vi "main 1.3.vi"() -> ()   [LabVIEW 2012]
uses:
  subvi/Newport ESP301/Newport ESP301.lvlib
  subvi/sp_manip.llb/sp_manip_lib.lvlib
  subvi/sp_manip.llb/tcp_gateway.lvlib
  subvi/PHOIBOS/DEFINITIONS/DEF_dev_type.ctl
  subvi/PHOIBOS/DEFINITIONS/DEF_dev_state.ctl
  <vilib>/Utility/file.llb/Write Delimited Spreadsheet (DBL).vi
  <vilib>/Analysis/NI_AALBase.lvlib
  <vilib>/Analysis/1siggen.llb/Ramp Pattern by Samples.vi
  <vilib>/Analysis/NI_AALPro.lvlib
  <vilib>/Analysis/_algsub.llb/Real Vector Norm.vi
  subvi/ZaberTSeries/ZaberTSeries.lvlib
  <vilib>/Utility/file.llb/Write Delimited Spreadsheet (string).vi
  <vilib>/Analysis/6fits.llb/Curve Fitting Criteria.ctl
  <vilib>/Instr/_visa.llb/VISA Configure Serial Port (Instr).vi
  <vilib>/DAQmx/create/channels.llb/DAQmx Create Channel (DI-Digital Input).vi
  <vilib>/Utility/file.llb/Read Delimited Spreadsheet (string).vi
panel:
  out "Pics L":i32=20
  out "Waveform Chart":dbl(graph)
  out "G2 X":cluster{dbl[], "Ramp Pattern":dbl[]}(graph)
  in  "reset every n pics":bool=TRUE
  in  "pics2avg":i32=50
  in  "abort acq.":bool
  out "G2 Y":cluster{dbl[], "Ramp Pattern":dbl[]}(graph)={[0.0, 0.0, 0.0, 0.0, 0.0, 0.0, 0.0, 0.0, 0.0, 0.0, 0.0, 0.0, 0.0, 0.0, 0.0, 0.0, 0.0, 0.0, 0.0, 0.0, 0.0, 0.0, 0.0, 0.0, 0.0, 0.0, 0.0, 0.0, 0.0, 0.0, 0.0, 0.0, 0.0, 0.0, 0.0, 0.0, 0.0, 0.0, 0.0, 0.0, 0.0, 0.0, 0.0, 0.0, 0.0, 0.0, 0.0, 0.0, 0.0, 0.0, 0.0, 0.0, 0.0, 0.0, 0.0, 0.0, 0.0, 0.0, 0.0, 0.0, 0.0, 0.0, 0.0, 0.0, 0.0, 0.0, 0.0, 0.0, 0.0, 0.0, 0.0, 0.0, 0.0, 0.0, 0.0, 0.0, 0.0, 0.0, 0.0, 0.0, 0.0, 0.0, 0.0, 0.0, 0.0, 0.0, 0.0, 0.0, 0.0, 0.0, 0.0, 0.0, 0.0, 0.0, 0.0, 0.0, 0.0, 0.0, 0.0, 0.0, 0.0, 0.0, 0.0, 0.0, 0.0, 0.0, 0.0, 0.0, 0.0, 0.0, 0.0, 0.0, 0.0, 0.0, 0.0, 0.0, 0.0, 0.0, 0.0, 0.0, 0.0, 0.0, 0.0, 0.0, 0.0, 0.0, 0.0, 0.0, 0.0, 0.0, 0.0, 0.0, 0.0, 0.0, 0.0, 0.0, 0.0, 0.0, 0.0, 0.0, 0.0, 0.0, 0.0, 0.0, 0.0, 0.0, 0.0, 0.0, 0.0, 0.0, 0.0, 0.0, 0.0, 0.0, 0.0, 0.0, 0.0, 0.0, 0.0, 0.0, 0.0, 0.0, 0.0, 0.0, 0.0, 0.0, 0.0, 0.0, 0.0, 0.0, 0.0, 0.0, 0.0, 0.0, 0.0, 0.0, 0.0, 0.0, 0.0, 0.0, 0.0, 0.0, 0.0, 0.0, 0.0, 0.0, 0.0, 0.0, 0.0, 0.0, 0.0, 0.0, 0.0, 0.0, 0.0, 0.0, 0.0, 0.0, 0.0, 0.0, 0.0, 0.0, 0.0, 0.0, 0.0, 0.0, 0.0, 0.0, 0.0, 0.0, 0.0, 0.0, 0.0, 0.0, 0.0, 0.0, 0.0, 0.0, 0.0, 0.0, 0.0, 0.0, 0.0, 0.0, 0.0, 0.0, 0.0, 0.0, 0.0, 0.0, 0.0, 0.0, 0.0, 0.0, 0.0, 0.0, 0.0, 0.0, 0.0, 0.0, 0.0, 0.0, 0.0, 0.0, 0.0, 0.0, 0.0, 0.0, 0.0, 0.0, 0.0, 0.0, 0.0, 0.0, 0.0, 0.0], "Ramp Pattern"=[0.0, 1.003921568627451, 2.007843137254902, 3.011764705882353, 4.015686274509804, 5.019607843137255, 6.023529411764706, 7.027450980392157, 8.031372549019608, 9.035294117647059, 10.03921568627451, 11.04313725490196, 12.047058823529412, 13.050980392156863, 14.054901960784314, 15.058823529411764, 16.062745098039215, 17.066666666666666, 18.070588235294117, 19.07450980392157, 20.07843137254902, 21.08235294117647, 22.08627450980392, 23.090196078431372, 24.094117647058823, 25.098039215686274, 26.101960784313725, 27.105882352941176, 28.109803921568627, 29.113725490196078, 30.11764705882353, 31.12156862745098, 32.12549019607843, 33.129411764705885, 34.13333333333333, 35.13725490196079, 36.141176470588235, 37.14509803921569, 38.14901960784314, 39.15294117647059, 40.15686274509804, 41.16078431372549, 42.16470588235294, 43.168627450980395, 44.17254901960784, 45.1764705882353, 46.180392156862744, 47.1843137254902, 48.188235294117646, 49.1921568627451, 50.19607843137255, 51.2, 52.20392156862745, 53.207843137254905, 54.21176470588235, 55.21568627450981, 56.219607843137254, 57.22352941176471, 58.227450980392156, 59.23137254901961, 60.23529411764706, 61.23921568627451, 62.24313725490196, 63.247058823529414, 64.25098039215686, 65.25490196078431, 66.25882352941177, 67.26274509803922, 68.26666666666667, 69.27058823529411, 70.27450980392157, 71.27843137254902, 72.28235294117647, 73.28627450980392, 74.29019607843138, 75.29411764705883, 76.29803921568627, 77.30196078431372, 78.30588235294118, 79.30980392156863, 80.31372549019608, 81.31764705882352, 82.32156862745099, 83.32549019607843, 84.32941176470588, 85.33333333333333, 86.33725490196079, 87.34117647058824, 88.34509803921569, 89.34901960784313, 90.3529411764706, 91.35686274509804, 92.36078431372549, 93.36470588235294, 94.3686274509804, 95.37254901960785, 96.37647058823529, 97.38039215686274, 98.3843137254902, 99.38823529411765, 100.3921568627451, 101.39607843137254, 102.4, 103.40392156862745, 104.4078431372549, 105.41176470588235, 106.41568627450981, 107.41960784313726, 108.4235294117647, 109.42745098039215, 110.43137254901961, 111.43529411764706, 112.43921568627451, 113.44313725490196, 114.44705882352942, 115.45098039215686, 116.45490196078431, 117.45882352941176, 118.46274509803922, 119.46666666666667, 120.47058823529412, 121.47450980392156, 122.47843137254903, 123.48235294117647, 124.48627450980392, 125.49019607843137, 126.49411764705883, 127.49803921568628, 128.50196078431372, 129.50588235294117, 130.50980392156862, 131.51372549019607, 132.51764705882354, 133.521568627451, 134.52549019607844, 135.52941176470588, 136.53333333333333, 137.53725490196078, 138.54117647058823, 139.54509803921567, 140.54901960784315, 141.5529411764706, 142.55686274509804, 143.5607843137255, 144.56470588235294, 145.5686274509804, 146.57254901960783, 147.57647058823528, 148.58039215686276, 149.5843137254902, 150.58823529411765, 151.5921568627451, 152.59607843137255, 153.6, 154.60392156862744, 155.6078431372549, 156.61176470588236, 157.6156862745098, 158.61960784313726, 159.6235294117647, 160.62745098039215, 161.6313725490196, 162.63529411764705, 163.6392156862745, 164.64313725490197, 165.64705882352942, 166.65098039215687, 167.65490196078431, 168.65882352941176, 169.6627450980392, 170.66666666666666, 171.6705882352941, 172.67450980392158, 173.67843137254903, 174.68235294117648, 175.68627450980392, 176.69019607843137, 177.69411764705882, 178.69803921568626, 179.7019607843137, 180.7058823529412, 181.70980392156864, 182.71372549019608, 183.71764705882353, 184.72156862745098, 185.72549019607843, 186.72941176470587, 187.73333333333332, 188.7372549019608, 189.74117647058824, 190.7450980392157, 191.74901960784314, 192.75294117647059, 193.75686274509803, 194.76078431372548, 195.76470588235293, 196.7686274509804, 197.77254901960785, 198.7764705882353, 199.78039215686275, 200.7843137254902, 201.78823529411764, 202.7921568627451, 203.79607843137254, 204.8, 205.80392156862746, 206.8078431372549, 207.81176470588235, 208.8156862745098, 209.81960784313725, 210.8235294117647, 211.82745098039214, 212.83137254901962, 213.83529411764707, 214.8392156862745, 215.84313725490196, 216.8470588235294, 217.85098039215686, 218.8549019607843, 219.85882352941175, 220.86274509803923, 221.86666666666667, 222.87058823529412, 223.87450980392157, 224.87843137254902, 225.88235294117646, 226.8862745098039, 227.89019607843136, 228.89411764705883, 229.89803921568628, 230.90196078431373, 231.90588235294118, 232.90980392156862, 233.91372549019607, 234.91764705882352, 235.92156862745097, 236.92549019607844, 237.9294117647059, 238.93333333333334, 239.93725490196078, 240.94117647058823, 241.94509803921568, 242.94901960784313, 243.95294117647057, 244.95686274509805, 245.9607843137255, 246.96470588235294, 247.9686274509804, 248.97254901960784, 249.9764705882353, 250.98039215686273, 251.98431372549018, 252.98823529411766, 253.9921568627451, 254.99607843137255, 256.0]}
  out "ETA":timestamp=timestamp(3553173084.423481 s since 1904-01-01) format="%<%H:%M:%S>T"
  out "acq. imgs":i32=20
  out "snap_prog":dbl(slide)=1.0 scale=0.0..1.0
  in  "BasePath":path=path "Z:/PESdata"
  in  "cam_liveavg":bool=TRUE caption="live average"
  out "cam_fps":dbl=19.770971874875205 caption="FPS" format="%.1g"
  out "sideimg":dbl[][](graph)
  in  "RunNumber":u16=50
  out "sum":dbl format="%#.2g"
  out "max":dbl
  out "mainimg":dbl[][](graph)
  out "ESP_con?":bool=TRUE caption="ESP301"
  out "phoib_con?":bool caption="PHOIBOS"
  out "manip_con?":bool=TRUE caption="manipulator"
  out "cam_con?":bool caption="camera"
  in  "main_close":bool
  in  "Tab Control":enum32{"live", "1D scan", "devices"}(tab)=enum."1D scan"
  in  "WP_rel +":bool
  in  "WP_rel -":bool
  in  "WP_delta":i32 caption="delta [steps]" min=0 step=1
  in  "WP_abs":bool
  in  "mirr_go":bool
  in  "ESP_opent0file":bool
  in  "mirr_rel":i32=20 caption="relative [steps]"
  in  "mirr_Y-":bool
  in  "mirr_Y+":bool
  in  "mirr_X+":bool
  in  "mirr_X-":bool
  in  "manip_deltas":dbl[](array[numeric])=[0.0, 0.0, 5.0, 0.0, 0.0, 0.0] caption="delta" format="%#.5g"
  in  "aq.mode":enum32{"Radio Selection 1", "Radio Selection 2"}(radio)=enum."Radio Selection 2"
  in  "dark avg":i32=100
  in  "cam_avgs":i32=20 caption="N"
  in  "ESP_delta":dbl caption="relative [mm]"
  in  "ESP_-":bool
  in  "ESP_+":bool
  in  "ESP_go":bool
  in  "ESP_dest_t":dbl=-12656.75602819869 caption="[fs]"
  in  "ESP_dest":dbl=25.0 caption="[mm]"
  in  "ESP_set_t0":bool
  in  "phoib_I_6s":dbl=3200.0
  in  "phoib_I_5s":dbl=1500.0
  in  "phoib_I_4s":dbl=4.558
  in  "phoib_I_3s":dbl=-7.0
  in  "phoib_I_2s":dbl=30.0
  in  "phoib_I_1s":dbl=18.0
  in  "phoib_standby":bool
  in  "phoib_set":bool
  out "phoib_I_6":dbl caption="Screen Voltage"
  out "phoib_I_5":dbl caption="Detctor Voltage"
  out "phoib_I_4":dbl caption="Work Function"
  out "phoib_I_3":dbl caption="Coil Current"
  out "phoib_I_2":dbl caption="Pass Energy"
  out "phoib_I_1":dbl caption="Kinetic Energy"
  out "Saved Positions":string[][](table)=[["ertwertwert", "-2.299945", "-2.030214", "38.900024", "50.000762", "0.000887", "-97.998082"], ["uztgugt", "-14.999451", "-13.638894", "442.380066", "13.998380", "-1.893758", "-76.305838"], ["asdf", "-14.999451", "-13.638894", "442.380066", "13.998380", "-1.893758", "-76.305838"], ["test3", "-14.999451", "-13.638894", "441.380066", "13.998380", "-1.893758", "-76.305838"]]
  in  "Save Pos":bool
  in  "Load":bool
  in  "Delete":bool
  in  "ManipRel +":bool
  in  "ManipRel -":bool
  in  "Move Abs":bool
  in  "stop manip":bool
  in  "dest":dbl[](array[numeric])=[-2.599774415331921, 2.6001372083008483, 64.7374267578125, 44.999124169862, 0.0008789063100814859, -80.99718876558107] caption="destination" format="%#.5g"
  out "axis":string[](array[string])=["x", "y", "z", "polar", "tilt", "azimut"]
  out "pos":dbl[](array[numeric])=[-1.8981328134268227, 1.9037561044451934, 84.7381591796875, 38.14189713860625, 0.0008789063100814859, -70.9987511093555] caption="position" format="%.5f"
  in  "ana_mode":T1(ring)=enum."WideAngleMode"
  in  "ana_voltrange":enum16{"3.5kV", "1.5kV", "400V", "100V", "10V"}(ring)=enum."400V"
  out "ESP_pos":dbl=31.74535 caption="Position"
  out "ESP_delay":dbl=45000.131390897084 caption="Delay"
  out "ESP_t0":dbl=25.0 caption="Time Zero @"
  out "phoib_I_7":dbl caption="Conversion Voltage"
  in  "phoib_I_7s":dbl=-26.0
  in  "phoib_I_8s":dbl=0.0039
  in  "phoib_I_9s":dbl=0.0039
  out "phoib_I_8":dbl caption="FD1"
  out "phoib_I_9":dbl caption="FD2"
  in  "gain":bool
  in  "cam_exp":u32=50 caption="exposure [ms]"
  in  "binning":u16(ring)=2 items=["X 1", "X 2", "X 4", "X 8"]
  in  "cam_dark?":bool=TRUE caption="subtract dark?"
  in  "cam_dark":bool
  in  "cam_saveimg":bool
  in  "e-size":u8
  in  "lower threshold":i32=50
  in  "count?":bool
  in  "ROI Left":i32=1
  in  "ROI Right":i32=43
  in  "ROI Top":i32=1
  in  "ROI Bottom":i32=33
  out "moving?":bool[](array[boolean])
  out "mirr_posX":i32=-9907 caption="X"
  out "mirr_posY":i32=-7260 caption="Y"
  in  "mirr_dest":i32[](array[numeric])=[-64, -2601]
  in  "WP_power.set":dbl caption="power set"
  out "WP_power":dbl caption="power"
  out "WP_deg":dbl caption="deg"
  out "WP_pos.steps":i32 caption="pos"
  out "Moving":bool
  in  "WP_angle.min":dbl caption="angle min"
  in  "WP_power.min":dbl caption="power min"
  in  "WP_power.max":dbl caption="power max"
  in  "clear delay table":bool
  in  "gauss fit":bool
  out "anglegraph":dbl[][](graph)
  out "intensitygraph":T2(graph)
  in  "scan_selector":T3(tab)
  in  "scan_manip_setstart":bool
  in  "scan_manip_start":dbl[](array[numeric])=[-2.6172862113166087, -0.009888298846365134, 68.5008544921875, -46.363686276590336, 11.108982061941884, -218.56360350415366] caption="start position" format="%#.5g"
  in  "scan_manip_deltas":dbl[](array[numeric])=[0.0, 0.0, 0.0, 0.0, 10.0, 0.0] caption="direction vector\n(gets normed)" format="%#.5g"
  in  "scan_mirr_start":i32[](array[numeric])=[-64, -2601]
  in  "scan_mirr_deltas":i32[](array[numeric])=[0, 0] caption="direction vector\n(gets normed)"
  in  "scan_mirr_setstart":bool
  in  "scan_volt_parameter":string(combo)="Kinetic Energy"
  in  "meas_iter":i32=60 caption="Iterations"
  out "duration [HH:MM:SS]":dbl=4512.494100093842 format="%<%H:%M:%S>t"
  out "disk [MB]":dbl=1028.5800000000002
  out "RAM [MB]":dbl=17.143
  out "total steps":i32=1860
  out "measpoints":i32=31
  in  "load delay table":bool
  in  "scan_go":bool
  in  "waypoints":string[][](table)=[["-100000", "5000"], ["50000", ""], ["", ""]]
  in  "stop after step":bool
  out "scan":dbl(slide)=0.967741935483871 scale=0.0..1.0
  out "iteration":dbl(slide)=0.03333333333333333 scale=0.0..1.0
  out "current scan":i32=30
  out "current iteration":i32=2
  in  "time/step [s]":dbl=2.426072096824646
  in  "stop after iteration":bool
  out "energygraph":dbl[][](graph)
  out "center":dbl
  in  "save delay table":bool
  in  "WP_init":bool
  in  "WP_release":bool
  in  "mirr_init":bool
  in  "mirr_release":bool
  in  "mirr_Y#":u8=2
  in  "manip_init":bool
  in  "manip_release":bool
  in  "phoib_init":bool
  in  "phoib_release":bool
  in  "ESP_init":bool
  in  "ESP_release":bool
  in  "ESP301 VISA":refnum<visa-resource-name>="COM8"
  in  "board number":i32
  in  "cam_init":bool
  in  "cam_release":bool
  out "cam_error":errorcluster
  out "phoib_error":errorcluster
  out "state":T4 items=["Off"=-1, "Standby"=0, "On"=1]
  in  "ESP Axis":i32=1 min=1 max=3
  out "error out":errorcluster
  out "error out 2":errorcluster
  out "mirr_Error":errorcluster
  in  "mirr_VISA":refnum<visa-resource-name>="COM7"
  in  "mirr_X#":u8=1
  in  "Operating mode\nHP & QE / HS & DiCam Pro":u32=1
  in  "Frame trigger \n(High Performance and QE only)":u16
  in  "WP_VISA":refnum<visa-resource-name>="COM8"
  in  "WP_baud":u32=9600
  out "WP_error":errorcluster
  # "camera"
  # "analyzer"
  # "manipulator"
  # "acquisition"
  # "delay stage"
  # "mirror"
  # "Position"
  # "Destination"
  # "watt pilot"
  # "- no settings -"
  # "waypoints are absolute values"
  # "- no settings -"
  # "waypoints are absolute values"
  # "X\nY\nZ\npolar\ntilt\nazimut"
  # "waypoint \"0\" is start position"
  # "X\nY"
  # "waypoint \"0\" is start position"
  # "waypoints are absolute values"
  # "camera"
  # "phoibos"
  # "ESP301"
  # "manipulator"
  # "mirror"
  # "0 = sequential\n1 = simultaneous"
  # "watt pilot"
  # "0 = internal\n1 = external rising\n2 = external falling"
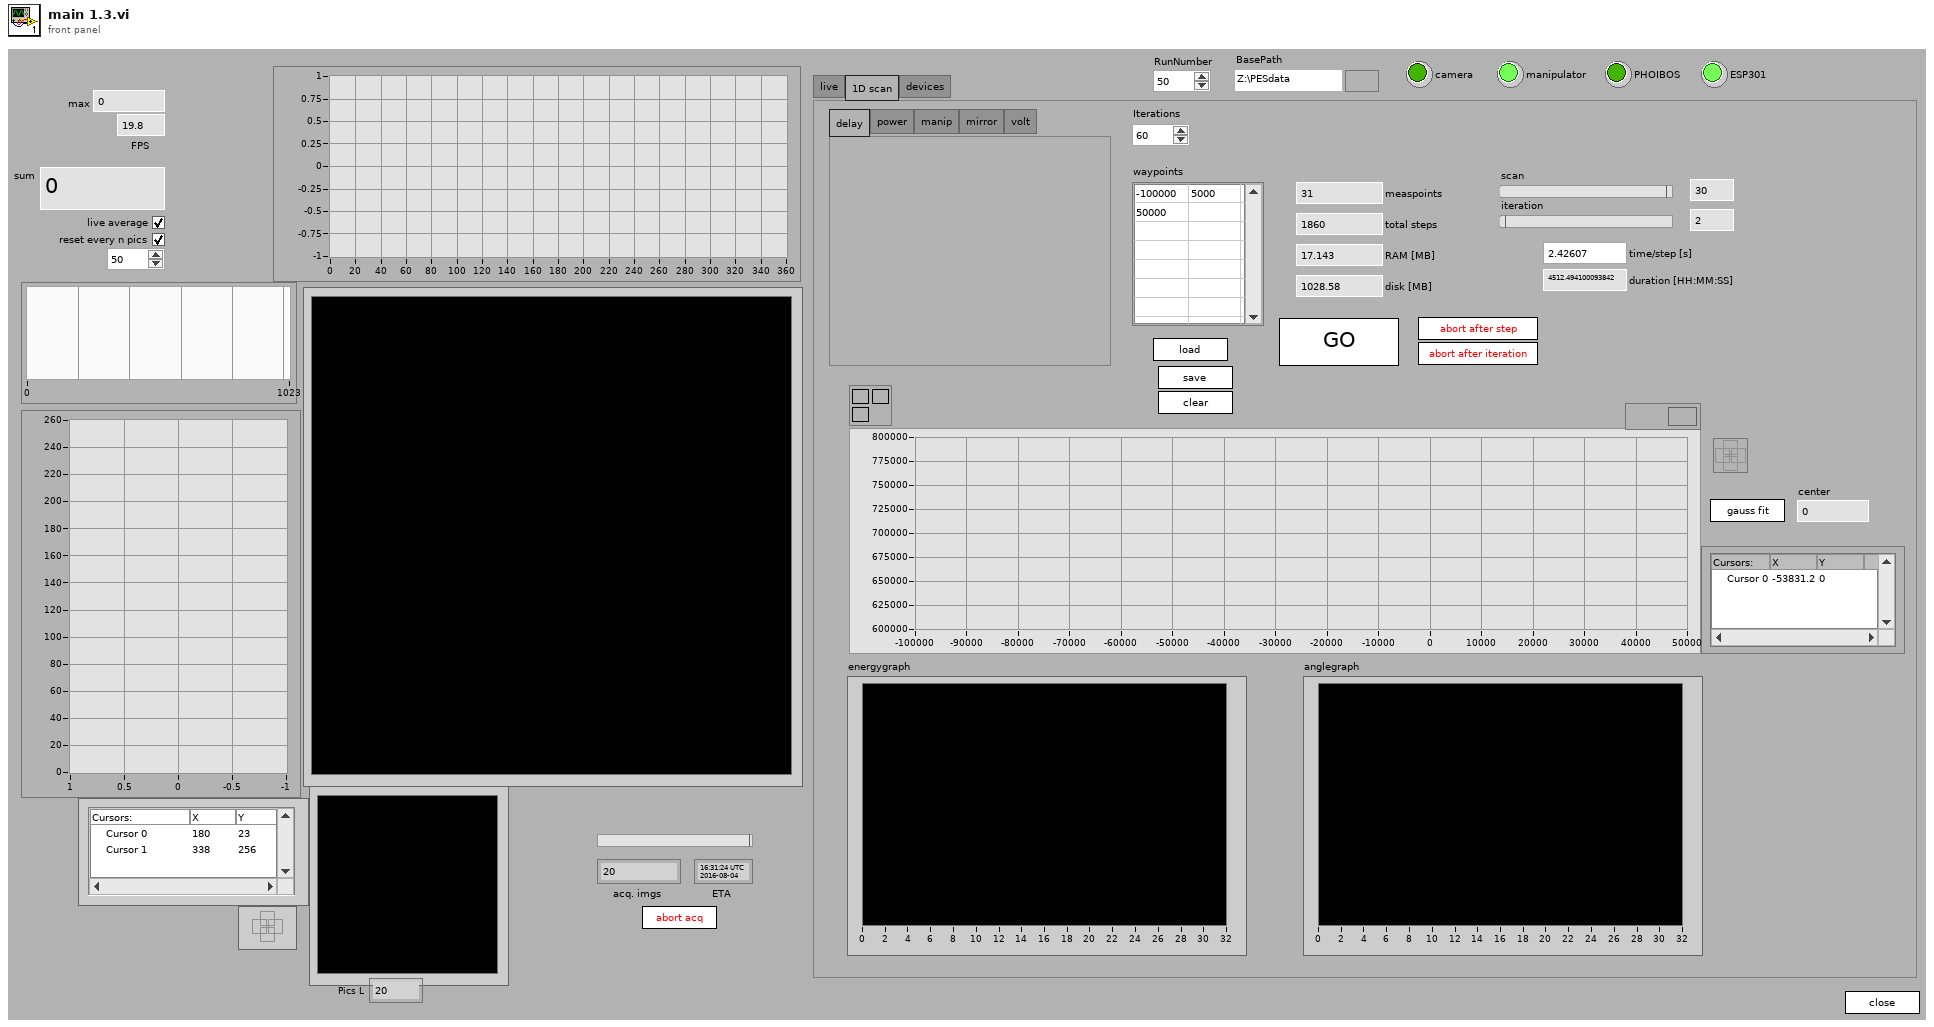
[diagram p1: front panel]
types:
  T1 = enum16{"HighMagnification", "MediumMagnification", "LowMagnification", "HighAngularDispersion", "MediumAngularDispersion", "LowAngularDispersion", "WideAngleMode", "LargeArea", "MediumArea", "SmallArea", "HighMagnification2", "SmallArea2", "ImagingMode"}
  T2 = cluster{"Array":dbl[], "Intensity Chart":dbl[]}[]
  T3 = enum32{"delay", "power", "manip", "mirror", "volt"}
  T4 = typedef "DEF_dev_state.ctl" = i32
  T5 = cluster{"queue out":refnum<queue>, "queue out":refnum<queue>, "queue out":refnum<queue>, "queue out":refnum<queue>, "queue out":refnum<queue>, "queue out":refnum<queue>}
  T6 = typedef "LVCursorListTypeDef.ctl" = cluster{"Name":string, "Color":u32, "Style":u8, "Point Style":u8, "Name Visible":bool, "Allow Drag":bool, "Cursor Mode":u32, "Plot":i32, "Index":i32, "Position":cluster{"X":dbl, "Y":dbl}, "X Scale":u32, "Y Scale":u32, "Watch Plots":i32[], "Watch All Plots":bool, "Plot Area":i32, "Label Offset":cluster{"X":dbl, "Y":dbl}}[]
  T7 = typedef "NI_AALPro.lvlib/Curve Fitting Criteria.ctl" = u16
  T8 = cluster{"Array":dbl[], "Best Gaussian Fit":dbl[]}
  T9 = cluster{"Array":dbl[], "Best Gaussian Fit":dbl[]}[]
  T10 = cluster{"Camera type":u32, "Operating mode\nHP & QE / HS & DiCam Pro ":u32, "Frame trigger \n(High Performance and QE only)":u16, "Sequence trigger":u16, "Low Light\n(QE only)":bool, "Gain":bool, "Horzontal\nbinning":u16, "Vertical\nbinning ":u16, "ROI Left":i32, "ROI Right":i32, "ROI Top":i32, "ROI Bottom":i32}
  T11 = cluster{"Name":string, "Color":u32, "Style":u8, "Point Style":u8, "Name Visible":bool, "Allow Drag":bool, "Cursor Mode":u32, "Plot":i32, "Index":i32, "Position":cluster{"X":dbl, "Y":dbl}, "X Scale":u32, "Y Scale":u32, "Watch Plots":i32[], "Watch All Plots":bool, "Plot Area":i32, "Label Offset":cluster{"X":dbl, "Y":dbl}}
  T12 = cluster{"mirr_X#":u8, "Command":u8, dbl, "Response Count":i32}
  T13 = cluster{"mirr_Y#":u8, "Command":u8, dbl, "Response Count":i32}
  T14 = cluster{i32, "Command":u8, i32, "Response Count":i32}
  T15 = cluster{"Axis_Name":string, "Axis_Type":string, "Axis_Position":dbl, "continous":bool, "moving":bool}[]
  T16 = typedef "DEF_dev_type.ctl" = enum32{"devA (analyzer)", "devD (detector)"}
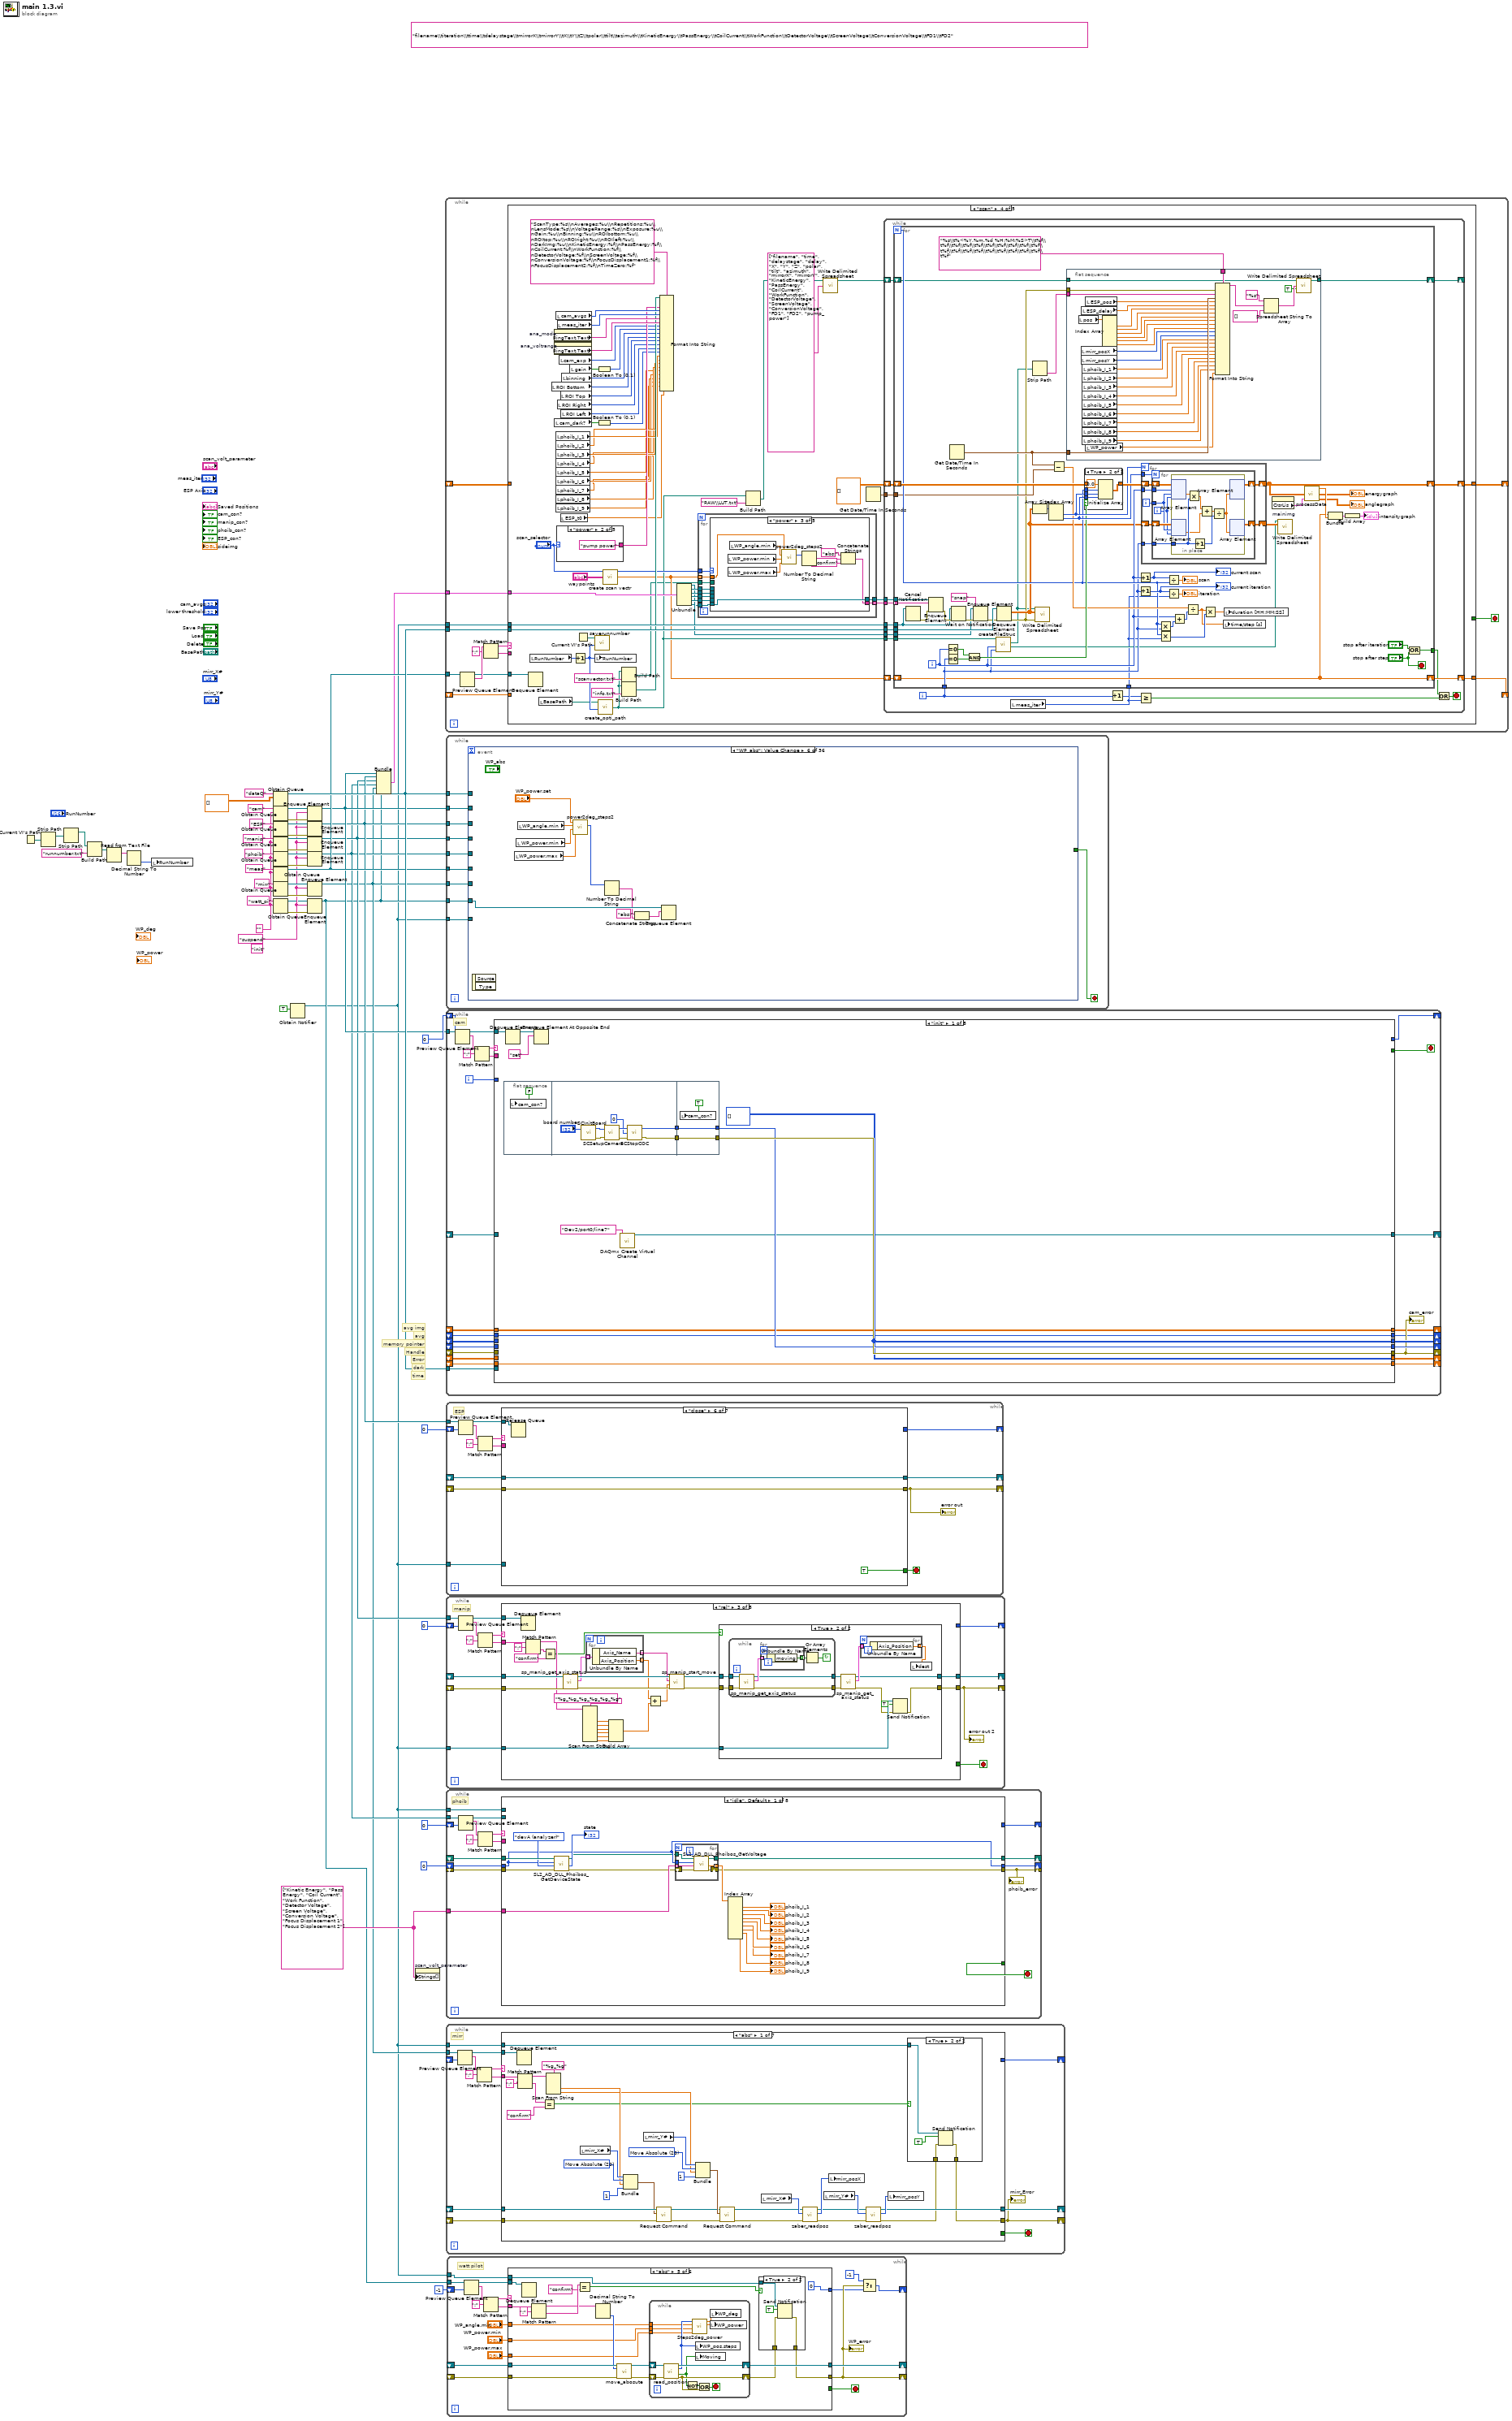
[diagram p0: block diagram]
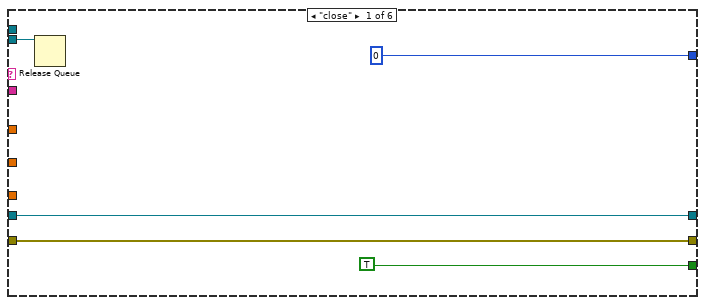
[diagram p2: hidden frame]
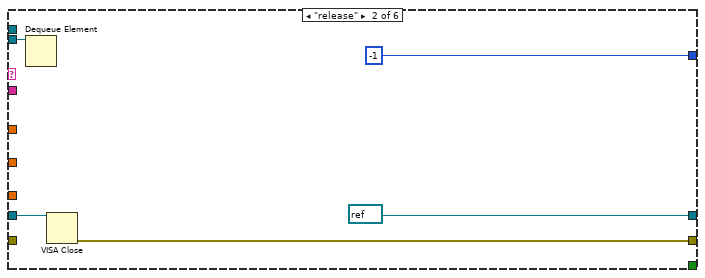
[diagram p3: hidden frame]
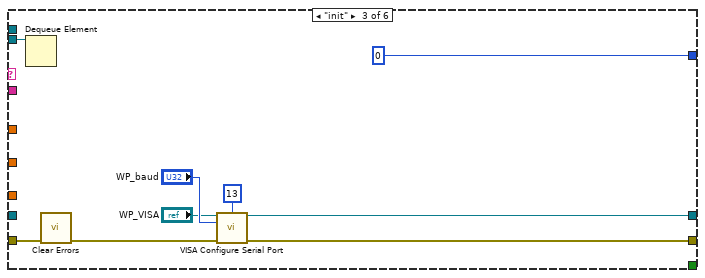
[diagram p4: hidden frame]
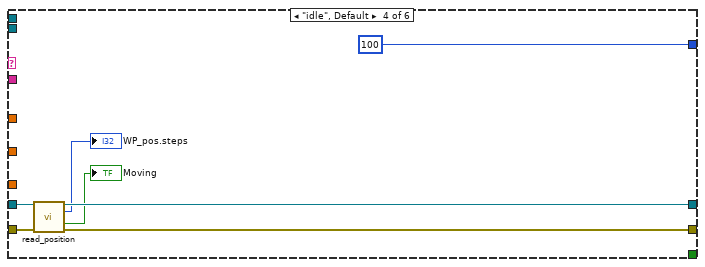
[diagram p5: hidden frame]
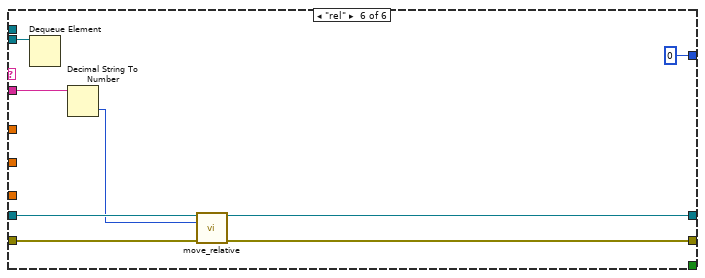
[diagram p7: hidden frame]
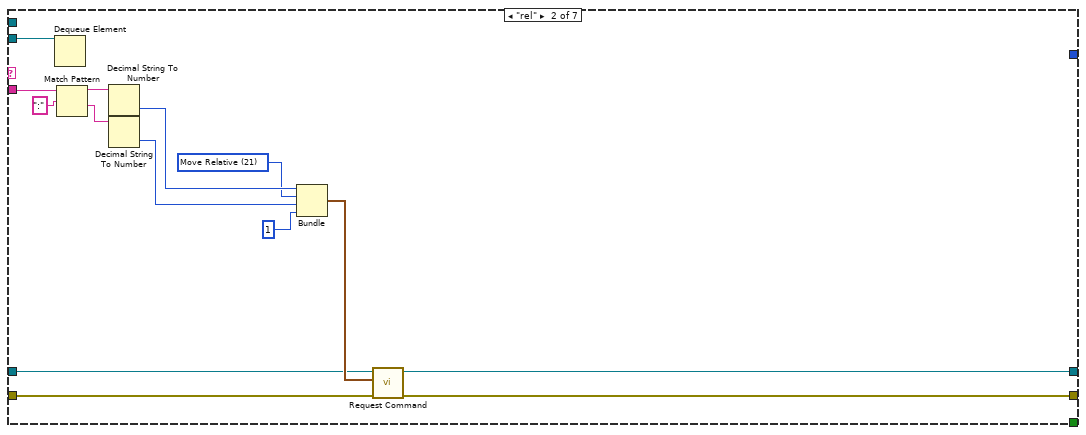
[diagram p9: hidden frame]
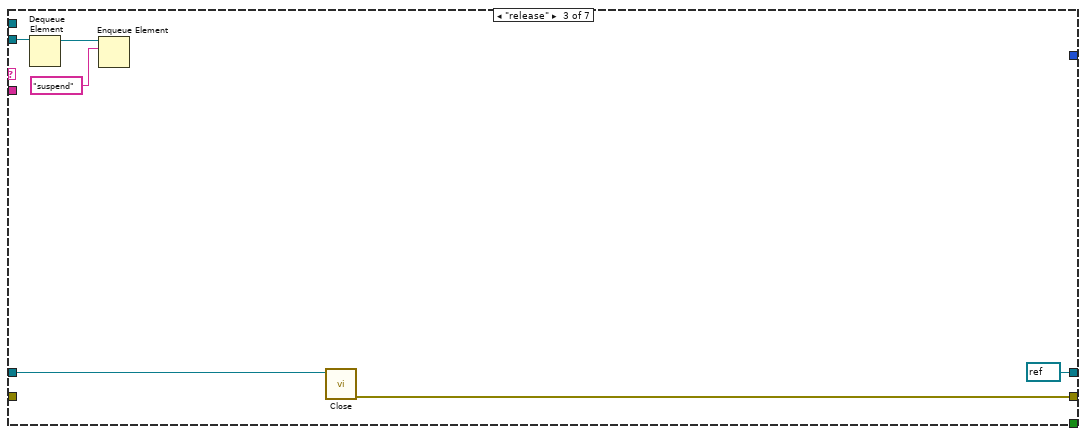
[diagram p10: hidden frame]
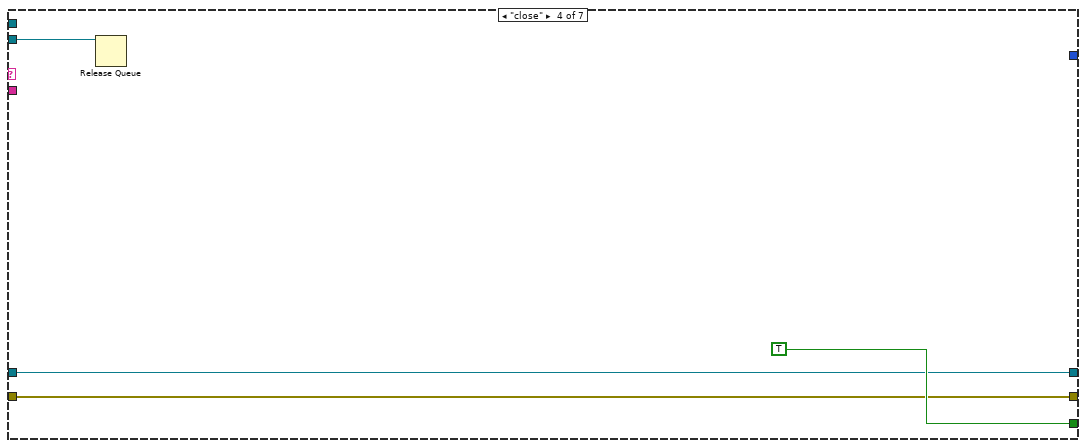
[diagram p11: hidden frame]
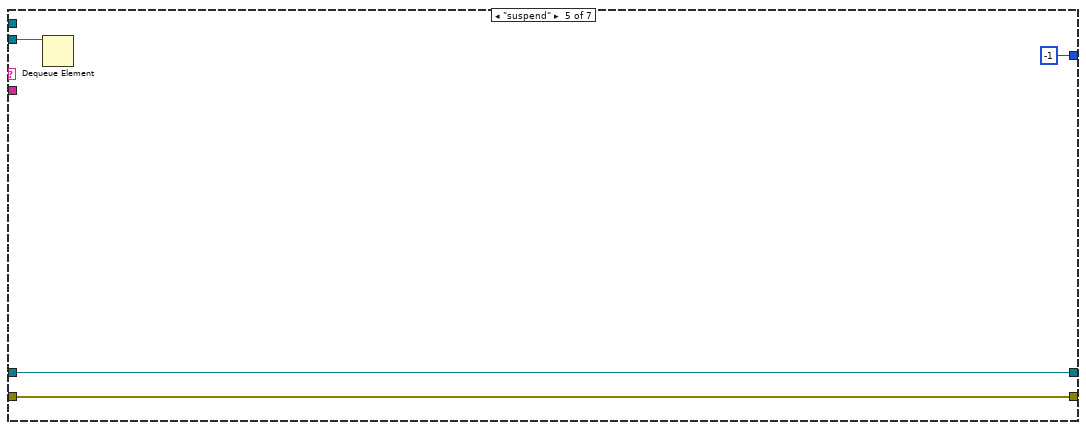
[diagram p12: hidden frame]
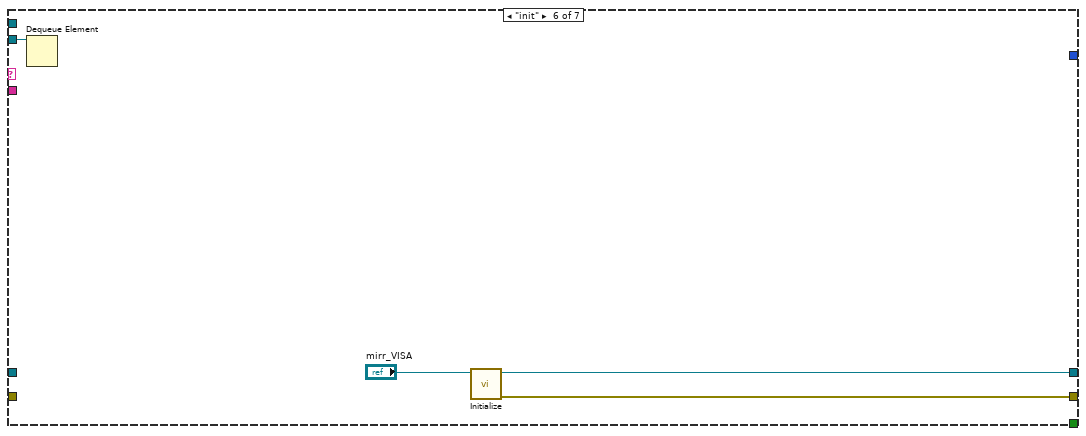
[diagram p13: hidden frame]
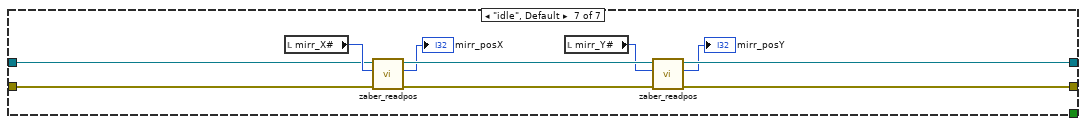
[diagram p14: hidden frame]
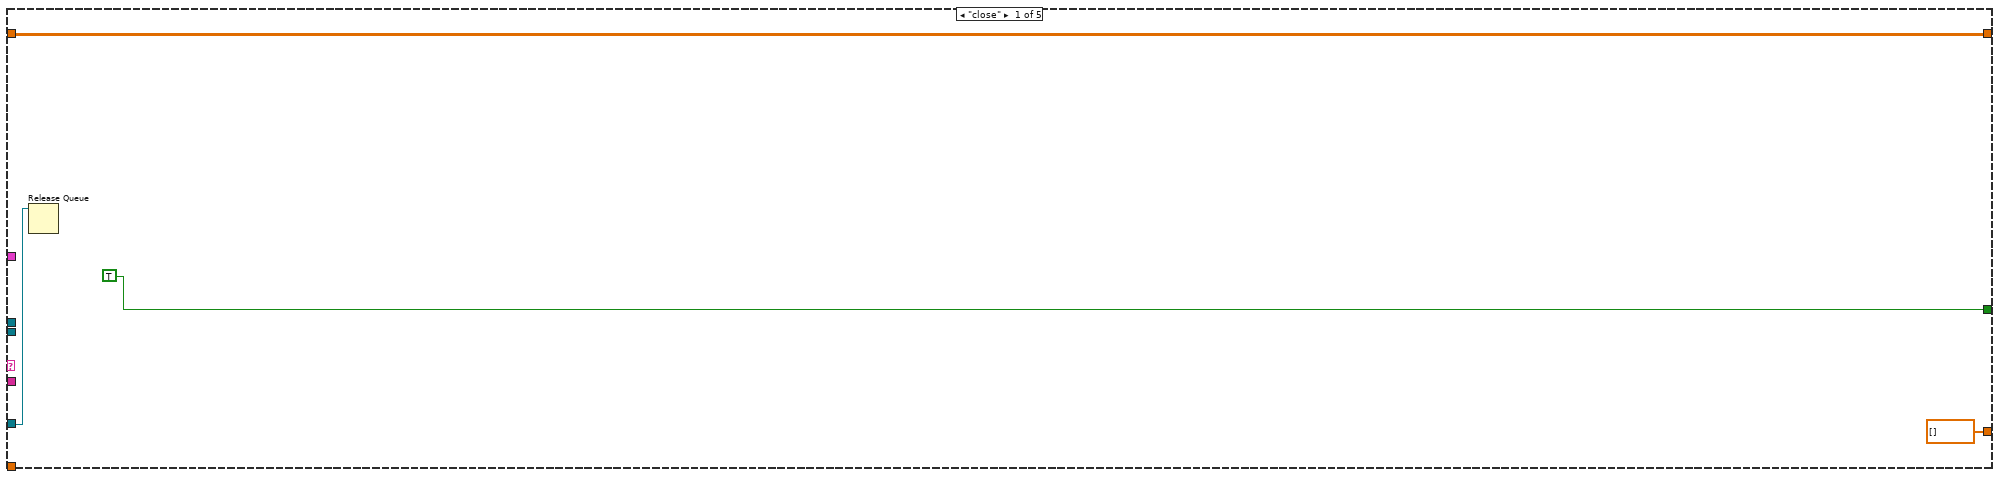
[diagram p15: hidden frame]
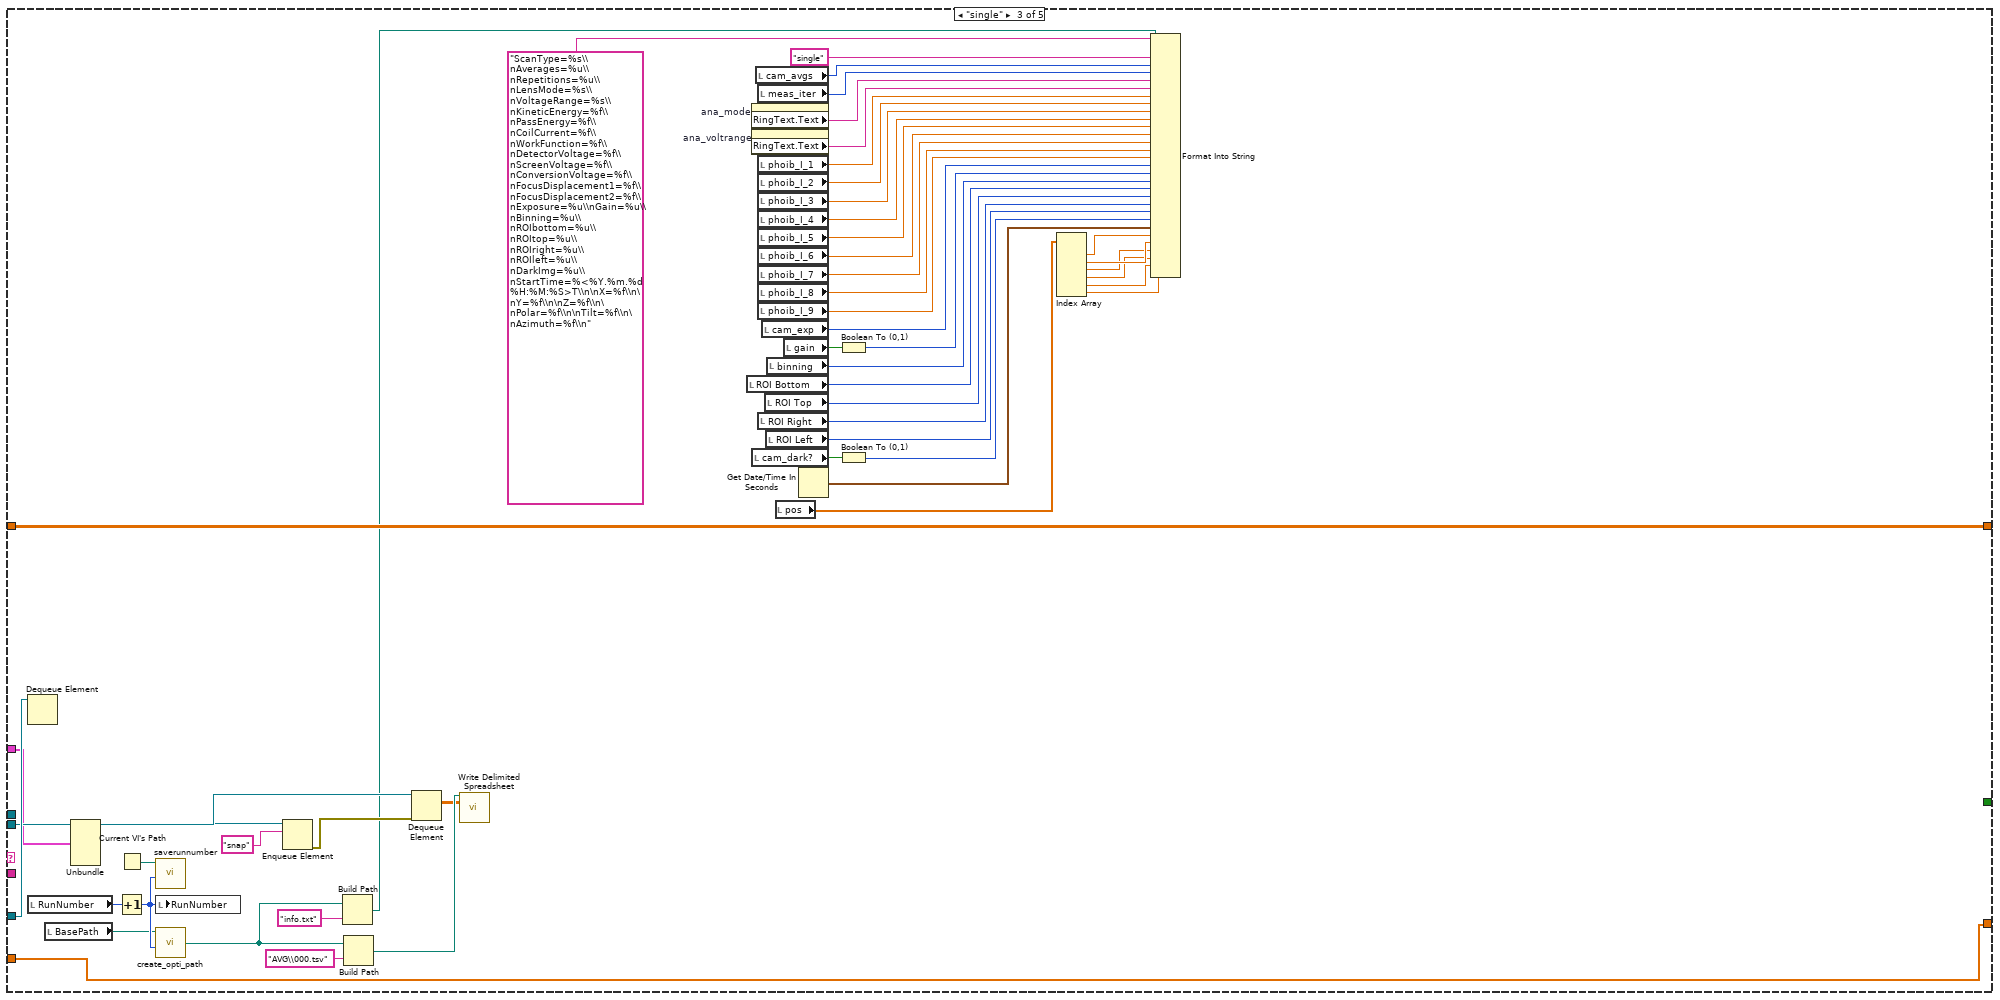
[diagram p17: hidden frame]
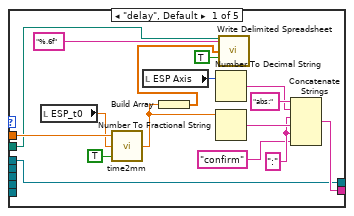
[diagram p19: hidden frame]
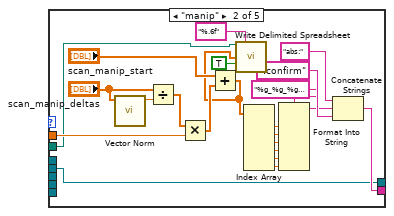
[diagram p20: hidden frame]
diagram:
  (unwired) "filename\\titeration\\ttime\\tdelaystage\\tmirrorX\\tmirrorY\\tX\\tY\\tZ\\tpolar\\ttilt\\tazimuth\\tKineticEnergy\\tPassEnergy\\tCoilCurrent\\tWorkFunction\\tDetectorVoltage\\tScreenVoltage\\tConversionVoltage\\tFD1\\tFD2"
  w15 = string[] ["Kinetic Energy", "Pass Energy", "Coil Current", "Work Function", "Detector Voltage", "Screen Voltage", "Conversion Voltage", "Focus Displacement 1", "Focus Displacement 2"]
  (unwired) "init" ("name (unnamed)")
  w7 = "suspend" ("name (unnamed)")
  w4 = "" ("name (unnamed)")
  # "avg img"
  # "avg"
  # "time"
  # "dark"
  # "Error"
  # "Handle"
  # "memory pointer"
  n1 = Current VI's Path() -> (path=w22:path)
  n2 = Strip Path(path=w22) -> (stripped path=w26:path)  [unwired: 1 out]
  n3 = Strip Path(path=w26) -> (stripped path=w27:path)  [unwired: 1 out]
  n4 = Build Path(base path=w27, name or relative path="runnumber.txt") -> (appended path=w24:path)
  n5 = Read from Text File(file (use dialog)=w24) -> (text=w25:string)  [unwired: 3 in, 3 out]
  n6 = Decimal String To Number(string=w25) -> (number=w9:i32)  [unwired: 2 in, 1 out]
  n7 = local write "RunNumber"(w9) -> ()
  n8 = Obtain Queue(name (unnamed)="dataQ", element data type=dbl[][] []) -> (queue out=w28:refnum<queue>)  [unwired: 3 in, 2 out]
  n9 = Obtain Queue(name (unnamed)="cam", element data type=w4) -> (queue out=w47:refnum<queue>, error out=w46:errorcluster)  [unwired: 3 in, 1 out]
  n10 = Obtain Queue(name (unnamed)="ESP", element data type=w4) -> (queue out=w44:refnum<queue>, error out=w45:errorcluster)  [unwired: 3 in, 1 out]
  n11 = Obtain Queue(name (unnamed)="manip", element data type=w4) -> (queue out=w41:refnum<queue>, error out=w40:errorcluster)  [unwired: 3 in, 1 out]
  n12 = Obtain Queue(name (unnamed)="phoib", element data type=w4) -> (queue out=w38:refnum<queue>, error out=w39:errorcluster)  [unwired: 3 in, 1 out]
  n13 = Obtain Queue(name (unnamed)="meas", element data type=w4) -> (queue out=w21:refnum<queue>)  [unwired: 3 in, 2 out]
  n14 = Obtain Queue(name (unnamed)="mirr", element data type=w4) -> (queue out=w13:refnum<queue>, error out=w12:errorcluster)  [unwired: 3 in, 1 out]
  n15 = Obtain Queue(name (unnamed)="watt_pi", element data type=w4) -> (queue out=w6:refnum<queue>, error out=w8:errorcluster)  [unwired: 3 in, 1 out]
  n16 = Obtain Notifier(notification data type=TRUE) -> (notifier out=w1:refnum<notifier>)  [unwired: 3 in, 2 out]
  n17 = Enqueue Element(queue=w47, element=w7, error in (no error)=w46) -> (queue out=w19:refnum<queue>)  [unwired: 1 in, 2 out]
  n18 = Enqueue Element(queue=w44, element=w7, error in (no error)=w45) -> (queue out=w18:refnum<queue>)  [unwired: 1 in, 2 out]
  n19 = Enqueue Element(queue=w41, element=w7, error in (no error)=w40) -> (queue out=w17:refnum<queue>)  [unwired: 1 in, 2 out]
  n20 = Enqueue Element(queue=w38, element=w7, error in (no error)=w39) -> (queue out=w16:refnum<queue>)  [unwired: 1 in, 2 out]
  n21 = Enqueue Element(queue=w13, element=w7, error in (no error)=w12) -> (queue out=w10:refnum<queue>)  [unwired: 1 in, 2 out]
  n22 = Enqueue Element(queue=w6, element=w7, error in (no error)=w8) -> (queue out=w2:refnum<queue>)  [unwired: 1 in, 2 out]
  n23 = Bundle("queue out"=w19, "queue out"=w18, "queue out"=w17, "queue out"=w16, "queue out"=w10, "queue out"=w2) -> (w20:T5)  [unwired: 1 in]
  n24 = property on="scan_volt_parameter" class="CmbBox"("Strings[]"=w15) -> ()  [unwired: 2 in, 2 out]
  n25 = while {
    tunnel: w28 -> [w62]
    tunnel: w21 -> [w59]
    tunnel: w20 -> [w55]
    shift-right: [w53] -> _
    shift-left: _ -> [w52]
    tunnel: w1 -> [w51]
    shift-right: [w50] -> _
    shift-left: _ -> [w49]
    stop <- w54 stop-if-true
    n26 = Preview Queue Element(queue=w59) -> (queue out=w56:refnum<queue>, element=w61:string)  [unwired: 2 in, 2 out]
    n27 = Match Pattern(string=w61, regular expression=":") -> (before substring=w58:string, after substring=w57:string)  [unwired: 1 in, 2 out]
    n28 = case shown="\"scan\"" w58 {
      tunnel: w62 -> [_ _ w118 w171 _]
      tunnel: w57 -> [_ _ _ _ _]
      tunnel: w56 -> [w66 _ w119 w167 w407]
      tunnel: [TRUE _ _ _ _] -> w54
      tunnel: w55 -> [_ _ w106 w147 _]
      tunnel: [w64 w68 w104 w169 w412] -> w53
      tunnel: w52 -> [w64 w68 w104 _ w412]
      tunnel: w51 -> [_ _ _ w168 _]
      tunnel: [dbl[] [] ("Array") w67 w76 w133 w409] -> w50
      tunnel: w49 -> [_ w67 w76 _ w409]
      frame "close" {
        n29 = Release Queue(queue=w66) -> ()  [unwired: 2 in, 3 out]
      }
      frame "idle", Default {
      }
      frame "single" {
        n30 = Dequeue Element(queue=w119) -> ()  [unwired: 2 in, 4 out]
        n31 = local read "RunNumber"() -> (w113:u16)
        n32 = local read "BasePath"() -> (w114:path)
        n33 = Unbundle(w106) -> ("queue out"=w105:refnum<queue>)  [unwired: 5 out]
        n34 = Increment(x=w113) -> (x+1=w115:u16)
        n35 = Current VI's Path() -> (path=w112:path)
        n36 = call "saverunnumber.vi"("RunNumber"=w115, "VI path"=w112) -> ()  [unwired: 10 in]
        n37 = local write "RunNumber"(w115) -> ()
        n38 = call "create_opti_path.vi"("RunNumber"=w115, "base path"=w114) -> ("Path"=w108:path)  [unwired: 2 in]
        n39 = Enqueue Element(queue=w105, element="snap" ("string")) -> (error out=w116:errorcluster)  [unwired: 2 in, 2 out]
        n40 = Build Path(base path=w108, name or relative path="info.txt") -> (appended path=w77:path)
        n41 = Build Path(base path=w108, name or relative path="AVG\\000.tsv") -> (appended path=w110:path)
        n42 = Dequeue Element(queue=w118, error in (no error)=w116) -> (element=w107:dbl[][])  [unwired: 1 in, 3 out]
        n43 = call-poly <vilib>:"Write Delimited Spreadsheet.vi"("file path (dialog if empty)"=w110, "2D data"=w107) -> ()  [unwired: 12 in, 2 out]
        n44 = local read "ROI Bottom"() -> (w84:i32)
        n45 = property on="ana_mode" class="Enum (strict)"() -> ("RingText.Text"=w99:string)  [unwired: 2 in, 2 out]
        n46 = property on="ana_voltrange" class="Enum (strict)"() -> ("RingText.Text"=w98:string)  [unwired: 2 in, 2 out]
        n47 = local read "cam_dark?"() -> (w80:bool)
        n48 = local read "cam_avgs"() -> (w101:i32)
        n49 = local read "meas_iter"() -> (w100:i32)
        n50 = local read "phoib_I_1"() -> (w97:dbl)
        n51 = local read "phoib_I_2"() -> (w96:dbl)
        n52 = local read "phoib_I_3"() -> (w95:dbl)
        n53 = local read "phoib_I_4"() -> (w94:dbl)
        n54 = local read "phoib_I_5"() -> (w93:dbl)
        n55 = local read "phoib_I_6"() -> (w92:dbl)
        n56 = local read "phoib_I_7"() -> (w91:dbl)
        n57 = local read "phoib_I_8"() -> (w90:dbl)
        n58 = local read "phoib_I_9"() -> (w89:dbl)
        n59 = local read "ROI Right"() -> (w82:i32)
        n60 = local read "cam_exp"() -> (w88:u32)
        n61 = local read "ROI Top"() -> (w83:i32)
        n62 = local read "ROI Left"() -> (w81:i32)
        n63 = local read "binning"() -> (w85:u16)
        n64 = local read "pos"() -> (w75:dbl[])
        n65 = local read "gain"() -> (w87:bool)
        n66 = Get Date/Time In Seconds() -> (seconds since 1Jan1904=w78:timestamp)
        n67 = Boolean To (0,1)(Boolean=w87) -> (0, 1=w86:i16)
        n68 = Boolean To (0,1)(Boolean=w80) -> (0, 1=w79:i16)
        n69 = Index Array(array=w75) -> (element #1=w74:dbl, element #2=w73:dbl, element #3=w72:dbl, element #4=w71:dbl, element #5=w70:dbl, element #6=w69:dbl)  [unwired: 6 in]
        n70 = Format Into String(format string="ScanType=%s\\nAverages=%u\\nRepetitions=%u\\nLensMode=%s\\nVoltageRange=%s\\nKineticEnergy=%f\\nPassEnergy=%f\\nCoilCurrent=%f\\nWorkFunction=%f\\nDetectorVoltage=%f\\nScreenVoltage=%f\\nConversionVoltage=%f\\nFocusDisplacement1=%f\\nFocusDisplacement2=%f\\nExposure=%u\\nGain=%u\\nBinning=%u\\nROIbottom=%u\\nROItop=%u\\nROIright=%u\\nROIleft=%u\\nDarkImg=%u\\nStartTime=%<%Y.%m.%d %H:%M:%S>T\\n\nX=%f\\n\nY=%f\\n\nZ=%f\\n\nPolar=%f\\n\nTilt=%f\\n\nAzimuth=%f\\n", initial string=w77, "single" ("input 1"), w101, w100, w99, w98, w97, w96, w95, w94, w93, w92, w91, w90, w89, w88, w86, w85, w84, w83, w82, w81, w79, w78, w74, w73, w72, w71, w70, w69) -> ()  [unwired: 1 in, 2 out]
      }
      frame "scan" {
        n71 = Dequeue Element(queue=w167) -> ()  [unwired: 2 in, 4 out]
        n72 = local read "RunNumber"() -> (w175:u16)
        n73 = local read "BasePath"() -> (w176:path)
        n74 = local read "ROI Bottom"() -> (w153:i32)
        n75 = property on="ana_mode" class="Enum (strict)"() -> ("RingText.Text"=w162:string)  [unwired: 2 in, 2 out]
        n76 = property on="ana_voltrange" class="Enum (strict)"() -> ("RingText.Text"=w161:string)  [unwired: 2 in, 2 out]
        n77 = local read "cam_dark?"() -> (w159:bool)
        n78 = local read "phoib_I_1"() -> (w131:dbl)
        n79 = local read "phoib_I_2"() -> (w130:dbl)
        n80 = local read "phoib_I_3"() -> (w129:dbl)
        n81 = local read "phoib_I_4"() -> (w128:dbl)
        n82 = local read "phoib_I_5"() -> (w127:dbl)
        n83 = local read "phoib_I_6"() -> (w126:dbl)
        n84 = local read "phoib_I_7"() -> (w125:dbl)
        n85 = local read "phoib_I_8"() -> (w124:dbl)
        n86 = local read "phoib_I_9"() -> (w123:dbl)
        n87 = local read "cam_avgs"() -> (w164:i32)
        n88 = case shown="\"power\"" "scan_selector" {
          tunnel: ["delay" ("input 1") "pump power" ("input 1") "manipulator" ("input 1") "mirror" ("input 1") "voltage" ("input 1")] -> w157
          frame "delay", Default {
          }
          frame "power" {
          }
          frame "manip" {
          }
          frame "mirror" {
          }
          frame "volt" {
          }
        }
        n89 = local read "meas_iter"() -> (w163:i32)
        n90 = local read "ROI Right"() -> (w151:i32)
        n91 = local read "cam_exp"() -> (w156:u32)
        n92 = local read "ROI Top"() -> (w152:i32)
        n93 = local read "ESP_t0"() -> (w122:dbl)
        n94 = local read "ROI Left"() -> (w150:i32)
        n95 = local read "binning"() -> (w154:u16)
        n96 = local read "gain"() -> (w160:bool)
        n97 = Increment(x=w175) -> (x+1=w177:u16)
        n98 = Current VI's Path() -> (path=w174:path)
        n99 = call "saverunnumber.vi"("RunNumber"=w177, "VI path"=w174) -> ()  [unwired: 10 in]
        n100 = local write "RunNumber"(w177) -> ()
        n101 = Boolean To (0,1)(Boolean=w160) -> (0, 1=w155:i16)
        n102 = Boolean To (0,1)(Boolean=w159) -> (0, 1=w149:i16)
        n103 = call "create_opti_path.vi"("RunNumber"=w177, "base path"=w176) -> ("Path"=w138:path)  [unwired: 2 in]
        n104 = call "create scan vectr.vi"("Table Control"="waypoints") -> ("Array"=w132:dbl[])
        n105 = Build Path(base path=w138, name or relative path="scanvector.txt") -> (appended path=w121:path)
        n106 = Build Path(base path=w138, name or relative path="info.txt") -> (appended path=w158:path)
        n107 = Format Into String(format string="ScanType:%s\\nAverages:%u\\nRepetitions:%u\\nLensMode:%s\\nVoltageRange:%s\\nExposure:%u\\nGain:%u\\nBinning:%u\\nROIbottom:%u\\nROItop:%u\\nROIright:%u\\nROIleft:%u\\nDarkImg:%u\\nKineticEnergy:%f\\nPassEnergy:%f\\nCoilCurrent:%f\\nWorkFunction:%f\\nDetectorVoltage:%f\\nScreenVoltage:%f\\nConversionVoltage:%f\\nFocusDisplacement1:%f\\nFocusDisplacement2:%f\\nTimeZero:%f", initial string=w158, w157, w164, w163, w162, w161, w156, w155, w154, w153, w152, w151, w150, w149, w131, w130, w129, w128, w127, w126, w125, w124, w123, w122) -> ()  [unwired: 1 in, 2 out]
        n108 = Unbundle(w147) -> ("queue out"=w139:refnum<queue>, "queue out"=w146:refnum<queue>, "queue out"=w145:refnum<queue>, "queue out"=w144:refnum<queue>, "queue out"=w143:refnum<queue>, "queue out"=w120:refnum<queue>)
        n109 = for {
          tunnel: w132 -> [w322] mode=indexing
          tunnel: [w321] -> w140 mode=indexing
          tunnel: [w320] -> w141
          tunnel: w146 -> [w319]
          tunnel: w145 -> [w318]
          tunnel: w144 -> [w317]
          tunnel: w143 -> [w316]
          tunnel: "scan_selector" -> [w315]
          tunnel: w121 -> [w314]
          tunnel: w120 -> [w313]
          n110 = case shown="\"power\"" w315 {
            tunnel: w322 -> [w330 w357 w363 w380 w390]
            tunnel: [w328 w345 w370 w377 w394] -> w320
            tunnel: [w334 w346 w361 w378 w395] -> w321
            tunnel: w319 -> [w328 _ _ _ _]
            tunnel: w318 -> [_ w345 _ _ _]
            tunnel: w317 -> [_ _ _ _ w394]
            tunnel: w316 -> [_ _ _ w377 _]
            tunnel: w314 -> [w323 w340 _ w374 w391]
            tunnel: w313 -> [_ _ w370 _ _]
            frame "delay", Default {
              w336 = ":" ("string")
              n111 = local read "ESP_t0"() -> (w329:dbl)
              n112 = call "time2mm.vi"("fs[1]/ps[0]"=TRUE, "Offset (mm)"=w329, "time"=w330) -> ("position (mm)"=w325:dbl)
              n113 = local read "ESP Axis"() -> (w333:i32)
              n114 = Build Array(w325) -> (w324:dbl[])
              n115 = Number To Decimal String(number=w333) -> (decimal integer string=w332:string)  [unwired: 1 in]
              n116 = Number To Fractional String(number=w325) -> (F-format string=w338:string)  [unwired: 3 in]
              n117 = call-poly <vilib>:"Write Delimited Spreadsheet.vi"("file path (dialog if empty)"=w323, "format (%.3f)"="%.6f", "1D data"=w324, "append to file? (F)"=TRUE) -> ()  [unwired: 10 in, 2 out]
              n118 = Concatenate Strings("abs:" ("string"), w332, w336, w338, w336, "confirm" ("string")) -> (w334:string)
            }
            frame "manip" {
              n119 = call-poly <vilib>:"Vector Norm.vi"("Input Vector"="scan_manip_deltas") -> ("norm"=w359:dbl)  [unwired: 9 in, 1 out]
              n120 = Divide(x="scan_manip_deltas", y=w359) -> (x/y=w358:dbl[])
              n121 = Multiply(x=w358, y=w357) -> (x*y=w343:dbl[])
              n122 = Add(x="scan_manip_start", y=w343) -> (x+y=w339:dbl[])
              n123 = call-poly <vilib>:"Write Delimited Spreadsheet.vi"("file path (dialog if empty)"=w340, "format (%.3f)"="%.6f", "1D data"=w339, "append to file? (F)"=TRUE) -> ()  [unwired: 10 in, 2 out]
              n124 = Index Array(array=w339) -> (element #1=w348:dbl, element #2=w349:dbl, element #3=w350:dbl, element #4=w351:dbl, element #5=w352:dbl, element #6=w353:dbl)  [unwired: 6 in]
              n125 = Format Into String(format string="%g_%g_%g_%g_%g_%g", w348, w349, w350, w351, w352, w353) -> (resulting string=w355:string)  [unwired: 2 in, 1 out]
              n126 = Concatenate Strings("abs:" ("string"), w355, ":confirm" ("string")) -> (w346:string)
            }
            frame "power" {
              n127 = local read "WP_power.min"() -> (w366:dbl)
              n128 = local read "WP_power.max"() -> (w365:dbl)
              n129 = local read "WP_angle.min"() -> (w367:dbl)
              n130 = call "power2deg_steps2.vi"("Max_power"=w365, "Min_power"=w366, "Min_angle"=w367, "Power"=w363) -> ("Steps"=w364:i32)  [unwired: 6 in, 1 out]
              n131 = Number To Decimal String(number=w364) -> (decimal integer string=w368:string)  [unwired: 1 in]
              n132 = Concatenate Strings("abs:" ("string"), w368, ":confirm" ("string")) -> (w361:string)
            }
            frame "mirror" {
              n133 = call-poly <vilib>:"Vector Norm.vi"("Input Vector"="scan_mirr_deltas") -> ("norm"=w388:dbl)  [unwired: 9 in, 1 out]
              n134 = Divide(x="scan_mirr_deltas", y=w388) -> (x/y=w387:dbl[])
              n135 = Multiply(x=w387, y=w380) -> (x*y=w376:dbl[])
              n136 = Add(x="scan_mirr_start", y=w376) -> (x+y=w373:dbl[])
              n137 = call-poly <vilib>:"Write Delimited Spreadsheet.vi"("file path (dialog if empty)"=w374, "format (%.3f)"="%.6f", "1D data"=w373, "append to file? (F)"=TRUE) -> ()  [unwired: 10 in, 2 out]
              n138 = Index Array(array=w373) -> (element #1=w383:dbl, element #2=w384:dbl)  [unwired: 2 in]
              n139 = Format Into String(format string="%g_%g", w383, w384) -> (resulting string=w386:string)  [unwired: 2 in, 1 out]
              n140 = Concatenate Strings("abs:" ("string"), w386, ":confirm" ("string")) -> (w378:string)
            }
            frame "volt" {
              n141 = local read "scan_volt_parameter"() -> (w398:string)
              n142 = Build Array(w390) -> (w389:dbl[])
              n143 = Number To Fractional String(number=w390) -> (F-format string=w396:string)  [unwired: 3 in]
              n144 = Concatenate Strings("setsgl:" ("string"), w398, ":" ("string"), w396) -> (w395:string)
              n145 = call-poly <vilib>:"Write Delimited Spreadsheet.vi"("file path (dialog if empty)"=w391, "format (%.3f)"="%.6f", "1D data"=w389, "append to file? (F)"=TRUE) -> ()  [unwired: 10 in, 2 out]
            }
          }
        }
        n146 = Build Path(base path=w138, name or relative path="RAW\\LUT.txt") -> (appended path=w136:path)
        n147 = call-poly <vilib>:"Write Delimited Spreadsheet.vi"("file path (dialog if empty)"=w136, "1D data"=string[] ["filename", "time", "delaystage", "delay", "X", "Y", "Z", "polar", "tilt", "azimuth", "mirrorX", "mirrorY", "KineticEnergy", "PassEnergy", "CoilCurrent", "WorkFunction", "DetectorVoltage", "ScreenVoltage", "ConversionVoltage", "FD1", "FD2", "pump_power"]) -> ("new file path (Not A Path if cancelled)"=w135:path)  [unwired: 12 in, 1 out]
        n148 = Get Date/Time In Seconds() -> (seconds since 1Jan1904=w148:timestamp)
        n149 = while {
          tunnel: w138 -> [w196]
          tunnel: w171 -> [w195]
          shift-right: [w194] -> w169
          shift-left: dbl[][][] [] -> [w193]
          tunnel: w168 -> [w192]
          tunnel: w148 -> [w191]
          tunnel: w141 -> [w190]
          tunnel: w140 -> [w189]
          tunnel: w139 -> [w188]
          shift-right: [w186] -> _
          shift-left: w135 -> [w187]
          shift-right: [w185] -> w133
          shift-left: w132 -> [w184]
          i -> [w183]
          stop <- w180 stop-if-true
          n150 = local read "meas_iter"() -> (w182:i32)
          n151 = for {
            N -> [w226]
            tunnel: w196 -> [w223]
            tunnel: w195 -> [w247]
            tunnel: w183 -> [w221]
            shift-right: [w236] -> w194
            shift-left: w193 -> [w243]
            tunnel: w192 -> [w238]
            tunnel: w191 -> [w225]
            tunnel: w190 -> [w217]
            tunnel: w189 -> [w216] mode=indexing
            tunnel: w188 -> [w215]
            shift-right: [w211] -> w186
            shift-left: w187 -> [w212]
            shift-right: [w207] -> w185
            shift-left: w184 -> [w207]
            tunnel: [w204] -> w179
            tunnel: w182 -> [w203]
            i -> [w222]
            stop <- "stop after step" stop-if-true
            n152 = Cancel Notification(0:w238) -> (11:w239:errorcluster)  [unwired: 1 in, 2 out]
            n153 = Enqueue Element(queue=w217, element=w216, error in (no error)=w239) -> (error out=w242:errorcluster)  [unwired: 1 in, 2 out]
            n154 = Equal To 0?(x=w222) -> (x = 0?=w246:bool)
            n155 = Equal To 0?(x=w221) -> (x = 0?=w245:bool)
            n156 = Get Date/Time In Seconds() -> (seconds since 1Jan1904=w213:timestamp)
            n157 = Wait on Notification(notifier=w238, error in (no error)=w242) -> (error out=w241:errorcluster)  [unwired: 2 in, 3 out]
            n158 = And(x=w246, y=w245) -> (x .and. y?=w244:bool)
            n159 = Enqueue Element(queue=w215, element="snap", error in (no error)=w241) -> (error out=w240:errorcluster)  [unwired: 1 in, 2 out]
            n160 = call "createFileStruc.vi"("i_iter"=w221, "i_delay"=w222, "meas_path"=w223) -> ("AVG file"=w218:path, "RAW file"=w209:path)  [unwired: 7 in]
            n161 = Dequeue Element(queue=w247, error in (no error)=w240) -> (element=w220:dbl[][], error out=w210:errorcluster)  [unwired: 1 in, 2 out]
            n162 = Strip Path(path=w209) -> (name=w208:string)  [unwired: 1 out]
            n163 = Array Size(array=w220) -> (size(s)=w251:i32[])
            n164 = call-poly <vilib>:"Write Delimited Spreadsheet.vi"("file path (dialog if empty)"=w209, "2D data"=w220, "error in (no error)"=w210) -> ()  [unwired: 11 in, 2 out]
            n165 = Index Array(array=w251) -> (element #1=w249:i32, element #2=w248:i32)  [unwired: 2 in]
            n166 = Subtract(x=w213, y=w225) -> (x-y=w229:dbl)
            n167 = flat-sequence {
              tunnel: "%s\\t%<%Y.%m.%d %H:%M:%S>T\\t%f\\t%f\\t%f\\t%f\\t%f\\t%f\\t%f\\t%f\\t%f\\t%f\\t%f\\t%f\\t%f\\t%f\\t%f\\t%f\\t%f\\t%f\\t%f\\t%f" -> [w282]
              tunnel: w213 -> [w281]
              tunnel: w212 -> [w258]
              tunnel: [w257] -> w211
              tunnel: w210 -> [w254]
              tunnel: w208 -> [w253]
              frame #0 {
                n168 = local read "pos"() -> (w283:dbl[])
                n169 = local read "mirr_posX"() -> (w270:i32)
                n170 = local read "mirr_posY"() -> (w271:i32)
                n171 = local read "ESP_delay"() -> (w263:dbl)
                n172 = local read "phoib_I_1"() -> (w272:dbl)
                n173 = local read "phoib_I_2"() -> (w273:dbl)
                n174 = local read "phoib_I_3"() -> (w274:dbl)
                n175 = local read "phoib_I_4"() -> (w275:dbl)
                n176 = local read "phoib_I_5"() -> (w276:dbl)
                n177 = local read "phoib_I_6"() -> (w277:dbl)
                n178 = local read "phoib_I_7"() -> (w278:dbl)
                n179 = local read "phoib_I_8"() -> (w279:dbl)
                n180 = local read "phoib_I_9"() -> (w280:dbl)
                n181 = local read "ESP_pos"() -> (w262:dbl)
                n182 = local read "WP_power"() -> (w252:dbl)
                n183 = Index Array(array=w283) -> (element #1=w264:dbl, element #2=w265:dbl, element #3=w266:dbl, element #4=w267:dbl, element #5=w268:dbl, element #6=w269:dbl)  [unwired: 6 in]
                n184 = Format Into String(format string=w282, error in=w254, w253, w281, w262, w263, w264, w265, w266, w267, w268, w269, w270, w271, w272, w273, w274, w275, w276, w277, w278, w279, w280, w252) -> (resulting string=w260:string)  [unwired: 1 in, 1 out]
                n185 = Spreadsheet String To Array(format string="%s", spreadsheet string=w260, array type (2D Dbl)=string[] []) -> (array=w256:string[])  [unwired: 1 in]
                n186 = call-poly <vilib>:"Write Delimited Spreadsheet.vi"("file path (dialog if empty)"=w258, "1D data"=w256, "append to file? (F)"=TRUE) -> ("new file path (Not A Path if cancelled)"=w257:path)  [unwired: 11 in, 1 out]
              }
            }
            n187 = case shown="True" w244 {
              tunnel: w226 -> [_ w289]
              tunnel: [w284 w287] -> w250
              tunnel: w243 -> [w284 _]
              tunnel: w249 -> [_ w286]
              tunnel: w248 -> [_ w285]
              frame False {
              }
              frame True {
                n188 = Initialize Array(0.0 ("element"), w289, w286, w285) -> (w287:dbl[][][])
              }
            }
            n189 = Increment(x=w222) -> (x+1=w233:i32)
            "current scan" <- w233
            n190 = Increment(x=w221) -> (x+1=w232:i32)
            "current iteration" <- w232
            n191 = for {
              N: w249 -> [_]
              tunnel: w222 -> [w296]
              shift-right: [w294] -> w236
              shift-left: w250 -> [w297]
              tunnel: w221 -> [w292]
              shift-right: [w291] -> w219
              shift-left: w220 -> [w293]
              tunnel: w248 -> [w290]
              i -> [w295]
              n192 = for {
                N: w290 -> [_]
                tunnel: w296 -> [w304]
                tunnel: w295 -> [w301]
                shift-right: [w303] -> w294
                shift-left: w297 -> [w305]
                tunnel: w292 -> [w299]
                shift-right: [w298] -> w291
                shift-left: w293 -> [w302]
                i -> [w300]
                n193 = in-place {
                  in-place-border: w299 -> [w311]
                  n194 = in-place-array #1(w305, w304, w301, w300) -> (w312:dbl)
                  n195 = in-place-array #2(w302, w301, w300) -> (w309:dbl)
                  n196 = Multiply(x=w312, y=w311) -> (x*y=w310:dbl)
                  n197 = Increment(x=w311) -> (x+1=w307:i32)
                  n198 = Add(x=w310, y=w309) -> (x+y=w308:dbl)
                  n199 = Divide(x=w308, y=w307) -> (x/y=w306:dbl)
                  n200 = in-place-array #1(w306) -> (w303:dbl[][][])  [unwired: 3 out]
                  n201 = in-place-array #2(w306) -> (w298:dbl[][])  [unwired: 2 out]
                }
              }
            }
            n202 = Multiply(x=w226, y=w221) -> (x*y=w228:i32)
            n203 = Multiply(x=w226, y=w203) -> (x*y=w224:i32)
            n204 = Divide(x=w233, y=w226) -> (x/y=→"scan":dbl)
            n205 = Divide(x=w232, y=w203) -> (x/y=→"iteration":dbl)
            n206 = Add(x=w222, y=w228) -> (x+y=w227:i32)
            n207 = Divide(x=w229, y=w227) -> (x/y=w199:dbl)
            n208 = Multiply(x=w199, y=w224) -> (x*y=w202:dbl)
            n209 = local write "time/step [s]"(w199) -> ()
            n210 = local write "duration [HH:MM:SS]"(w202) -> ()
            n211 = property on="mainimg" class="IntGraph (strict)"() -> ("CrsrLis"=w235:T6)  [unwired: 2 in, 2 out]
            n212 = call-poly <vilib>:"Write Delimited Spreadsheet.vi"("file path (dialog if empty)"=w218, "2D data"=w219) -> ()  [unwired: 12 in, 2 out]
            n213 = call "processData.vi"("Cursor List"=w235, "data in"=w236) -> ("Angle Chart"=→"anglegraph":dbl[][], "Energy Chart"=→"energygraph":dbl[][], "Intensity Chart"=w234:dbl[])  [unwired: 1 in]
            n214 = Bundle("Array"=w207, "Intensity Chart"=w234) -> (w198:cluster{"Array":dbl[], "Intensity Chart":dbl[]})  [unwired: 1 in]
            n215 = Build Array(w198) -> (→"intensitygraph":T2)
            n216 = Or(x="stop after iteration", y="stop after step") -> (x .or. y?=w204:bool)
          }
          n217 = Increment(x=w183) -> (x+1=w181:i32)
          n218 = Greater Or Equal?(x=w181, y=w182) -> (x >= y?=w178:bool)
          n219 = Or(x=w179, y=w178) -> (x .or. y?=w180:bool)
        }
      }
      frame "refresh" {
        n220 = Dequeue Element(queue=w407) -> ()  [unwired: 2 in, 4 out]
        n221 = property on="mainimg" class="IntGraph (strict)"() -> ("CrsrLis"=w413:T6)  [unwired: 2 in, 2 out]
        n222 = call "processData.vi"("Cursor List"=w413, "data in"=w412) -> ("Angle Chart"=w410:dbl[][], "Energy Chart"=w411:dbl[][], "Intensity Chart"=w408:dbl[])  [unwired: 1 in]
        n223 = Bundle("Array"=w409, "Intensity Chart"=w408) -> (w406:cluster{"Array":dbl[], "Intensity Chart":dbl[]})  [unwired: 1 in]
        n224 = Build Array(w406) -> (w405:T2)
        n225 = local write "energygraph"(w411) -> ()
        n226 = local write "intensitygraph"(w405) -> ()
        n227 = local write "anglegraph"(w410) -> ()
      }
    }
  }
  n228 = while {
    tunnel: w19 -> [w422]
    tunnel: w18 -> [w421]
    tunnel: w17 -> [w420]
    tunnel: w16 -> [w419]
    tunnel: w21 -> [w417]
    tunnel: w28 -> [w418]
    tunnel: w1 -> [w416]
    tunnel: w10 -> [w415]
    tunnel: w2 -> [w414]
    stop <- w423 stop-if-true
    n229 = event shown="[5] \"WP_abs\": Value Change" {
      selector: _ -> [_ _ _ _ _ _ _ _ _ _ _ _ _ _ _ _ _ _ _ _ _ _ _ _ _ _ _ _ _ _ _ _ _ _ _ _]
      dyn-events: _ -> [_ _ _ _ _ _ _ _ _ _ _ _ _ _ _ _ _ _ _ _ _ _ _ _ _ _ _ _ _ _ _ _ _ _ _ _]
      timeout: _ -> [_ _ _ _ _ _ _ _ _ _ _ _ _ _ _ _ _ _ _ _ _ _ _ _ _ _ _ _ _ _ _ _ _ _ _ _]
      tunnel: [_ TRUE _ _ _ _ _ _ _ _ _ _ _ _ _ _ _ _ _ _ _ _ _ _ _ _ _ _ _ _ _ _ _ _ _ _] -> w423
      tunnel: w422 -> [_ w441 w452 _ _ _ _ _ _ _ _ w500 w502 _ _ _ _ _ _ _ _ _ _ _ _ _ _ _ _ _ _ _ _ _ _ _]
      tunnel: w421 -> [_ w440 _ w456 _ _ _ _ _ _ _ _ _ _ _ _ _ _ _ _ _ _ _ _ w585 _ _ w607 _ _ _ _ _ _ _ _]
      tunnel: w420 -> [_ w439 _ _ _ _ _ w484 _ _ _ _ _ _ _ _ _ _ _ _ w552 w568 _ w577 _ _ _ _ _ _ _ _ _ _ _ _]
      tunnel: w419 -> [_ w438 _ _ _ _ _ _ w490 w496 w497 _ _ _ _ _ _ _ _ _ _ _ _ _ _ _ _ _ _ _ _ _ _ _ _ _]
      tunnel: w418 -> [_ w445 _ _ _ _ _ _ _ _ _ _ _ _ _ _ _ _ _ _ _ _ _ _ _ _ _ _ _ _ _ _ _ _ _ _]
      tunnel: w417 -> [_ w437 _ _ _ _ _ _ _ _ _ _ _ w504 w506 _ _ _ _ _ _ _ _ _ _ _ _ _ _ _ _ _ _ w630 _ _]
      tunnel: w416 -> [_ w444 _ _ _ _ _ _ _ _ _ _ _ _ _ _ _ _ _ _ _ _ _ _ _ _ _ _ _ _ _ _ _ _ _ _]
      tunnel: w415 -> [_ w436 _ _ _ _ _ _ _ _ _ _ _ _ _ _ _ w530 _ _ _ _ _ _ _ _ _ _ _ _ _ _ _ _ w632 w653]
      tunnel: w414 -> [_ w428 _ _ w462 w474 w482 _ _ _ _ _ _ _ _ _ _ _ _ _ _ _ _ _ _ _ _ _ _ _ _ _ _ _ _ _]
      event Timeout {
        n230 = event-data() -> ()  [unwired: 1 in, 1 out]
      }
      event "main_close": Value Change {
        w425 = "close" ("element")
        w424 = "release" ("element")
        n231 = event-data() -> ()  [unwired: 1 in, 1 out]
        n232 = Flush Queue(queue=w441) -> (queue out=w435:refnum<queue>)  [unwired: 1 in, 2 out]
        n233 = Flush Queue(queue=w440) -> (queue out=w434:refnum<queue>)  [unwired: 1 in, 2 out]
        n234 = Flush Queue(queue=w439) -> (queue out=w433:refnum<queue>)  [unwired: 1 in, 2 out]
        n235 = Flush Queue(queue=w438) -> (queue out=w432:refnum<queue>)  [unwired: 1 in, 2 out]
        n236 = Flush Queue(queue=w437) -> (queue out=w431:refnum<queue>)  [unwired: 1 in, 2 out]
        n237 = Flush Queue(queue=w436) -> (queue out=w430:refnum<queue>)  [unwired: 1 in, 2 out]
        n238 = Flush Queue(queue=w428) -> (queue out=w427:refnum<queue>)  [unwired: 1 in, 2 out]
        n239 = Release Notifier(notifier=w444) -> ()  [unwired: 2 in, 3 out]
        n240 = Release Queue(queue=w445) -> ()  [unwired: 2 in, 3 out]
        n241 = Enqueue Element(queue=w435, element=w424) -> (queue out=w449:refnum<queue>)  [unwired: 2 in, 2 out]
        n242 = Enqueue Element(queue=w434, element=w424) -> (queue out=w448:refnum<queue>)  [unwired: 2 in, 2 out]
        n243 = Enqueue Element(queue=w433, element=w424) -> (queue out=w447:refnum<queue>)  [unwired: 2 in, 2 out]
        n244 = Enqueue Element(queue=w432, element=w424) -> (queue out=w446:refnum<queue>)  [unwired: 2 in, 2 out]
        n245 = Enqueue Element(queue=w430, element=w424) -> (queue out=w443:refnum<queue>, error out=w442:errorcluster)  [unwired: 2 in, 1 out]
        n246 = Enqueue Element(queue=w427, element=w424) -> (queue out=w426:refnum<queue>, error out=w429:errorcluster)  [unwired: 2 in, 1 out]
        n247 = Enqueue Element(queue=w449, element=w425) -> ()  [unwired: 2 in, 3 out]
        n248 = Enqueue Element(queue=w448, element=w425) -> ()  [unwired: 2 in, 3 out]
        n249 = Enqueue Element(queue=w447, element=w425) -> ()  [unwired: 2 in, 3 out]
        n250 = Enqueue Element(queue=w446, element=w425) -> ()  [unwired: 2 in, 3 out]
        n251 = Enqueue Element(queue=w431, element=w425) -> ()  [unwired: 2 in, 3 out]
        n252 = Enqueue Element(queue=w443, element=w425, error in (no error)=w442) -> ()  [unwired: 1 in, 3 out]
        n253 = Enqueue Element(queue=w426, element=w425, error in (no error)=w429) -> ()  [unwired: 1 in, 3 out]
      }
      event "cam_release", "cam_init": Value Change {
        n254 = event-data() -> ()  [unwired: 1 in, 2 out]
        n255 = Select(t="init" ("name (unnamed)"), s="cam_init", f="release" ("name (unnamed)")) -> (s? t:f=w451:string)
        n256 = Enqueue Element(queue=w452, element=w451) -> ()  [unwired: 2 in, 3 out]
      }
      event "ESP_release", "ESP_init": Value Change {
        n257 = event-data() -> ()  [unwired: 1 in, 2 out]
        n258 = Select(t="init" ("name (unnamed)"), s="ESP_init", f="release" ("name (unnamed)")) -> (s? t:f=w460:string)
        n259 = Enqueue Element(queue=w456, element=w460) -> ()  [unwired: 2 in, 3 out]
      }
      event "WP_init", "WP_release": Value Change {
        n260 = event-data() -> ()  [unwired: 1 in, 2 out]
        n261 = Select(t="init" ("name (unnamed)"), s="WP_init", f="release" ("name (unnamed)")) -> (s? t:f=w465:string)
        n262 = Enqueue Element(queue=w462, element=w465) -> ()  [unwired: 2 in, 3 out]
      }
      event "WP_abs": Value Change {
        n263 = event-data() -> ()  [unwired: 1 in, 2 out]
        n264 = local read "WP_power.max"() -> (w468:dbl)
        n265 = local read "WP_power.min"() -> (w469:dbl)
        n266 = local read "WP_angle.min"() -> (w470:dbl)
        n267 = call "power2deg_steps2.vi"("Max_power"=w468, "Min_power"=w469, "Min_angle"=w470, "Power"="WP_power.set") -> ("Steps"=w466:i32)  [unwired: 6 in, 1 out]
        n268 = Number To Decimal String(number=w466) -> (decimal integer string=w471:string)  [unwired: 1 in]
        n269 = Concatenate Strings("abs:" ("string"), w471) -> (w472:string)
        n270 = Enqueue Element(queue=w474, element=w472) -> ()  [unwired: 2 in, 3 out]
      }
      event "WP_rel -", "WP_rel +": Value Change {
        n271 = event-data() -> ()  [unwired: 1 in, 2 out]
        n272 = Negate(x="WP_delta") -> (-x=w477:i32)
        n273 = Select(t="WP_delta", s="WP_rel +", f=w477) -> (s? t:f=w475:i32)
        n274 = Number To Decimal String(number=w475) -> (decimal integer string=w479:string)  [unwired: 1 in]
        n275 = Concatenate Strings("rel:" ("string"), w479) -> (w481:string)
        n276 = Enqueue Element(queue=w482, element=w481) -> ()  [unwired: 2 in, 3 out]
      }
      event "manip_init", "manip_release": Value Change {
        n277 = event-data() -> ()  [unwired: 1 in, 2 out]
        n278 = Flush Queue(queue=w484) -> (queue out=w483:refnum<queue>)  [unwired: 1 in, 2 out]
        n279 = Select(t="init" ("name (unnamed)"), s="manip_init", f="release" ("name (unnamed)")) -> (s? t:f=w486:string)
        n280 = Enqueue Element(queue=w483, element=w486) -> ()  [unwired: 2 in, 3 out]
      }
      event "phoib_release", "phoib_init": Value Change {
        n281 = event-data() -> ()  [unwired: 1 in, 2 out]
        n282 = Flush Queue(queue=w490) -> (queue out=w489:refnum<queue>)  [unwired: 1 in, 2 out]
        n283 = Select(t="init" ("name (unnamed)"), s="phoib_init", f="release" ("name (unnamed)")) -> (s? t:f=w492:string)
        n284 = Enqueue Element(queue=w489, element=w492) -> ()  [unwired: 2 in, 3 out]
      }
      event "phoib_standby": Value Change {
        n285 = event-data() -> ()  [unwired: 1 in, 2 out]
        n286 = Enqueue Element(queue=w496, element="standby") -> ()  [unwired: 2 in, 3 out]
      }
      event "phoib_set": Value Change {
        n287 = event-data() -> ()  [unwired: 1 in, 2 out]
        n288 = Enqueue Element(queue=w497, element="set") -> ()  [unwired: 2 in, 3 out]
      }
      event "cam_dark": Value Change {
        n289 = event-data() -> ()  [unwired: 1 in, 2 out]
        n290 = Enqueue Element(queue=w500, element="dark") -> ()  [unwired: 2 in, 3 out]
      }
      event "ROI Left", "ROI Right", "ROI Top", "ROI Bottom", "cam_exp", "binning", "gain": Value Change {
        n291 = event-data() -> ()  [unwired: 1 in, 1 out]
        n292 = Enqueue Element(queue=w502, element="set") -> ()  [unwired: 2 in, 3 out]
      }
      event "cam_saveimg": Value Change {
        n293 = event-data() -> ()  [unwired: 1 in, 1 out]
        n294 = Enqueue Element(queue=w504, element="single") -> ()  [unwired: 2 in, 3 out]
      }
      event "scan_go": Value Change {
        n295 = event-data() -> ()  [unwired: 1 in, 1 out]
        n296 = Enqueue Element(queue=w506, element="scan") -> ()  [unwired: 2 in, 3 out]
      }
      event "meas_iter", "waypoints": Value Change {
        n297 = event-data() -> ()  [unwired: 1 in, 6 out]
        n298 = local read "waypoints"() -> (w518:string[][])
        n299 = local read "meas_iter"() -> (w512:i32)
        n300 = local read "binning"() -> (w515:u16)
        n301 = call "create scan vectr.vi"("Table Control"=w518) -> ("Array"=w517:dbl[])
        n302 = Index Array(array=dbl[] [8.79, 2.2, 0.553, 0.138], index=w515) -> (element=w511:dbl)
        n303 = Array Size(array=w517) -> (size(s)=w514:i32)
        "measpoints" <- w514
        n304 = Multiply(x=w514, y=w512) -> (x*y=w509:i32)
        "total steps" <- w509
        n305 = Multiply(x=w509, y="time/step [s]") -> (x*y=→"duration [HH:MM:SS]":dbl)
        n306 = Multiply(x=w514, y=w511) -> (x*y=→"RAM [MB]":dbl)
        n307 = Multiply(x=w509, y=w511) -> (x*y=→"disk [MB]":dbl)
      }
      event "gauss fit": Value Change {
        w528 = T7 2 items=["Least Square", "Least Absolute Residual", "Bisquare"] ("method")
        n308 = event-data() -> ()  [unwired: 1 in, 6 out]
        n309 = local read "intensitygraph"() -> (w520:T2)
        n310 = Index Array(array=w520) -> (element=w519:cluster{"Array":dbl[], "Intensity Chart":dbl[]})  [unwired: 1 in]
        n311 = Unbundle(w519) -> ("Array"=w525:dbl[], "Intensity Chart"=w526:dbl[])
        n312 = call <vilib>:"Gaussian Peak Fit.vi"("Y"=w526, "X"=w525, "method"=w528) -> ("Best Gaussian Fit"=w524:dbl[], "center"=→"center":dbl)  [unwired: 6 in, 5 out]
        n313 = Bundle("Array"=w525, "Intensity Chart"=w526) -> (w523:cluster{"Array":dbl[], "Intensity Chart":dbl[]})  [unwired: 1 in]
        n314 = Bundle("Array"=w525, "Best Gaussian Fit"=w524) -> (w522:T8)  [unwired: 1 in]
        n315 = Build Array(w523, w522) -> (w521:T9)
        n316 = local write "intensitygraph"(w521) -> ()
      }
      event "mirr_go": Value Change {
        n317 = event-data() -> ()  [unwired: 1 in, 1 out]
        n318 = Index Array(array="mirr_dest") -> (element #1=w535:i32, element #2=w534:i32)  [unwired: 2 in]
        n319 = Format Into String(format string="%g_%g", w535, w534) -> (resulting string=w532:string)  [unwired: 2 in, 1 out]
        n320 = Concatenate Strings("abs:" ("string"), w532) -> (w529:string)
        n321 = Enqueue Element(queue=w530, element=w529) -> ()  [unwired: 2 in, 3 out]
      }
      event "scan_manip_setstart": Value Change {
        n322 = event-data() -> ()  [unwired: 1 in, 1 out]
        n323 = local read "pos"() -> (w537:dbl[])
        n324 = local write "scan_manip_start"(w537) -> ()
      }
      event "scan_mirr_setstart": Value Change {
        n325 = event-data() -> ()  [unwired: 1 in, 1 out]
        n326 = local read "mirr_posX"() -> (w540:i32)
        n327 = local read "mirr_posY"() -> (w539:i32)
        n328 = Build Array(w540, w539) -> (w538:i32[])
        n329 = local write "scan_mirr_start"(w538) -> ()
      }
      event "Move Abs": Value Change {
        n330 = event-data() -> ()  [unwired: 1 in, 1 out]
        n331 = Index Array(array="dest") -> (element #1=w550:dbl, element #2=w549:dbl, element #3=w548:dbl, element #4=w547:dbl, element #5=w546:dbl, element #6=w545:dbl)  [unwired: 6 in]
        n332 = Format Into String(format string="%g_%g_%g_%g_%g_%g", w550, w549, w548, w547, w546, w545) -> (resulting string=w543:string)  [unwired: 2 in, 1 out]
        n333 = Concatenate Strings("abs:" ("string"), w543) -> (w542:string)
        n334 = Enqueue Element(queue=w552, element=w542) -> ()  [unwired: 2 in, 3 out]
      }
      event "ManipRel +", "ManipRel -": Value Change {
        n335 = event-data() -> ()  [unwired: 1 in, 2 out]
        n336 = Negate(x="manip_deltas") -> (-x=w556:dbl[])
        n337 = Select(t="manip_deltas", s="ManipRel +", f=w556) -> (s? t:f=w554:dbl[])
        n338 = Index Array(array=w554) -> (element #1=w560:dbl, element #2=w561:dbl, element #3=w562:dbl, element #4=w563:dbl, element #5=w564:dbl, element #6=w565:dbl)  [unwired: 6 in]
        n339 = Format Into String(format string="%g_%g_%g_%g_%g_%g", w560, w561, w562, w563, w564, w565) -> (resulting string=w567:string)  [unwired: 2 in, 1 out]
        n340 = Concatenate Strings("rel:" ("string"), w567, ":confirm" ("string")) -> (w558:string)
        n341 = Enqueue Element(queue=w568, element=w558) -> ()  [unwired: 2 in, 3 out]
      }
      event "RunNumber": Value Change {
        n342 = event-data() -> ()  [unwired: 1 in, 6 out]
        n343 = Current VI's Path() -> (path=w575:path)
        n344 = local read "RunNumber"() -> (w571:u16)
        n345 = Strip Path(path=w575) -> (stripped path=w573:path)  [unwired: 1 out]
        n346 = Strip Path(path=w573) -> (stripped path=w572:path)  [unwired: 1 out]
        n347 = Build Path(base path=w572, name or relative path="runnumber.txt") -> (appended path=w569:path)
        n348 = Number To Decimal String(number=w571) -> (decimal integer string=w570:string)  [unwired: 1 in]
        n349 = Write to Text File(file (use dialog)=w569, text=w570) -> ()  [unwired: 2 in, 3 out]
      }
      event "stop manip": Value Change {
        n350 = event-data() -> ()  [unwired: 1 in, 1 out]
        n351 = Enqueue Element(queue=w577, element="stop") -> ()  [unwired: 2 in, 3 out]
      }
      event "ESP_go": Value Change {
        w579 = ":" ("string")
        n352 = event-data() -> ()  [unwired: 1 in, 1 out]
        n353 = local read "ESP Axis"() -> (w578:i32)
        n354 = Number To Decimal String(number=w578) -> (decimal integer string=w581:string)  [unwired: 1 in]
        n355 = Number To Fractional String(number="ESP_dest") -> (F-format string=w580:string)  [unwired: 3 in]
        n356 = Concatenate Strings("abs:" ("string"), w581, w579, w580, w579) -> (w584:string)
        n357 = Enqueue Element(queue=w585, element=w584) -> ()  [unwired: 2 in, 3 out]
      }
      event "ESP_set_t0": Value Change {
        n358 = event-data() -> ()  [unwired: 1 in, 1 out]
        n359 = Current VI's Path() -> (path=w596:path)
        n360 = Strip Path(path=w596) -> (stripped path=w594:path)  [unwired: 1 out]
        n361 = Strip Path(path=w594) -> (stripped path=w593:path)  [unwired: 1 out]
        n362 = local read "ESP_pos"() -> (w595:dbl)
        "ESP_t0" <- w595
        n363 = Number To Fractional String(number=w595) -> (F-format string=w588:string)  [unwired: 3 in]
        n364 = Build Path(base path=w593, name or relative path="t0.txt") -> (appended path=w590:path)
        n365 = Get Date/Time In Seconds() -> (seconds since 1Jan1904=w592:timestamp)
        n366 = Format Date/Time String(time format string (%c)="%Y.%m.%d %H:%M", seconds (now)=w592) -> (date/time string=w589:string)  [unwired: 1 in]
        n367 = Build Array(w589, w588) -> (w587:string[])
        n368 = call-poly <vilib>:"Write Delimited Spreadsheet.vi"("file path (dialog if empty)"=w590, "1D data"=w587, "append to file? (F)"=TRUE) -> ()  [unwired: 11 in, 2 out]
      }
      event "ESP_opent0file": Value Change {
        n369 = event-data() -> ()  [unwired: 1 in, 6 out]
        n370 = Current VI's Path() -> (path=w600:path)
        n371 = Strip Path(path=w600) -> (stripped path=w599:path)  [unwired: 1 out]
        n372 = Strip Path(path=w599) -> (stripped path=w601:path)  [unwired: 1 out]
        n373 = call <vilib>:"System Exec.vi"("wait until completion? (T)"=FALSE, "working directory"=w601, "command line"="notepad t0.txt") -> ()  [unwired: 5 in, 4 out]
      }
      event "ESP_+", "ESP_-": Value Change {
        n374 = event-data() -> ()  [unwired: 1 in, 6 out]
        n375 = local read "ESP Axis"() -> (w603:i32)
        n376 = Negate(x="ESP_delta") -> (-x=w610:dbl)
        n377 = Select(t="ESP_delta", s="ESP_+", f=w610) -> (s? t:f=w608:dbl)
        n378 = Number To Decimal String(number=w603) -> (decimal integer string=w606:string)  [unwired: 1 in]
        n379 = Number To Fractional String(number=w608) -> (F-format string=w604:string)  [unwired: 3 in]
        n380 = Concatenate Strings("rel:" ("string"), w606, ":" ("string"), w604) -> (w613:string)
        n381 = Enqueue Element(queue=w607, element=w613) -> ()  [unwired: 2 in, 3 out]
      }
      event "ESP_dest": Value Change {
        n382 = event-data() -> ()  [unwired: 1 in, 6 out]
        n383 = local read "ESP_dest"() -> (w617:dbl)
        n384 = local read "ESP_t0"() -> (w616:dbl)
        n385 = call "mm2time.vi"("fs?"=TRUE ("fs[1]/ps[0]"), "Offset (mm)"=w616, "distance (mm)"=w617) -> ("time in fs/ps seconds"=w614:dbl)
        n386 = local write "ESP_dest_t"(w614) -> ()
      }
      event "ESP_dest_t": Value Change {
        n387 = event-data() -> ()  [unwired: 1 in, 1 out]
        n388 = local read "ESP_t0"() -> (w620:dbl)
        n389 = call "time2mm.vi"("fs[1]/ps[0]"=TRUE, "Offset (mm)"=w620, "time"="ESP_dest_t") -> ("position (mm)"=w618:dbl)
        n390 = local write "ESP_dest"(w618) -> ()
      }
      event "load delay table": Value Change {
        n391 = event-data() -> ()  [unwired: 1 in, 6 out]
        n392 = call-poly <vilib>:"Read Delimited Spreadsheet.vi"() -> ("all rows"=w623:string[][], "error out"=w622:errorcluster)  [unwired: 10 in, 4 out]
        n393 = case shown="No Error" w622 {
          tunnel: w623 -> [w624 _]
          frame No Error {
            n394 = local write "waypoints"(w624) -> ()
          }
          frame Error {
          }
        }
      }
      event "save delay table": Value Change {
        n395 = event-data() -> ()  [unwired: 1 in, 6 out]
        n396 = local read "waypoints"() -> (w625:string[][])
        n397 = call-poly <vilib>:"Write Delimited Spreadsheet.vi"("2D data"=w625) -> ()  [unwired: 13 in, 2 out]
      }
      event "clear delay table": Value Change {
        w627 = 0 ("dimension size")
        n398 = event-data() -> ()  [unwired: 1 in, 6 out]
        n399 = Initialize Array("", w627, w627) -> (w626:string[][])
        n400 = local write "waypoints"(w626) -> ()
      }
      event "mainimg": Cursor Release {
        n401 = event-data() -> ()  [unwired: 1 in, 1 out]
        n402 = Enqueue Element(queue=w630, element="refresh") -> ()  [unwired: 2 in, 3 out]
      }
      event "mirr_init", "mirr_release": Value Change {
        n403 = event-data() -> ()  [unwired: 1 in, 6 out]
        n404 = Flush Queue(queue=w632) -> (queue out=w633:refnum<queue>)  [unwired: 1 in, 2 out]
        n405 = Select(t="init" ("name (unnamed)"), s="mirr_init", f="release" ("name (unnamed)")) -> (s? t:f=w634:string)
        n406 = Enqueue Element(queue=w633, element=w634) -> ()  [unwired: 2 in, 3 out]
      }
      event "mirr_X-", "mirr_X+", "mirr_Y+", "mirr_Y-": Value Change {
        n407 = event-data() -> ()  [unwired: 1 in, 1 out]
        n408 = local read "mirr_X#"() -> (w644:u8)
        n409 = local read "mirr_Y#"() -> (w643:u8)
        n410 = Or(x="mirr_X+", y="mirr_X-") -> (x .or. y?=w645:bool)
        n411 = Or(x="mirr_X-", y="mirr_Y-") -> (x .or. y?=w651:bool)
        n412 = Negate(x="mirr_rel") -> (-x=w650:i32)
        n413 = Select(t=w644, s=w645, f=w643) -> (s? t:f=w642:u8)
        n414 = Select(t=w650, s=w651, f="mirr_rel") -> (s? t:f=w639:i32)
        n415 = Number To Decimal String(number=w642) -> (decimal integer string=w641:string)  [unwired: 1 in]
        n416 = Number To Decimal String(number=w639) -> (decimal integer string=w638:string)  [unwired: 1 in]
        n417 = Concatenate Strings("rel:" ("string"), w641, ":" ("string"), w638) -> (w637:string)
        n418 = Enqueue Element(queue=w653, element=w637) -> ()  [unwired: 2 in, 3 out]
      }
    }
  }
  n419 = while {
    tunnel: w19 -> [w680]
    shift-right: [w674] -> _
    shift-left: _ -> [w673]
    shift-right: [w672] -> _
    shift-left: _ -> [w670]
    shift-right: [w671] -> _
    shift-left: _ -> [w669]
    shift-right: [w666] -> _
    shift-left: 0 -> [w667]
    shift-right: [w665] -> _
    shift-left: _ -> [w664]
    shift-right: [w663] -> _
    shift-left: _ -> [w662]
    tunnel: w28 -> [w661]
    shift-right: [w660] -> _
    shift-left: _ -> [w659]
    shift-right: [w657] -> _
    shift-left: _ -> [w656]
    shift-right: [w655] -> _
    shift-left: _ -> [w654]
    i -> [w658]
    stop <- w668 stop-if-true
    # "cam"
    n420 = Preview Queue Element(queue=w680, timeout in ms (-1)=w667) -> (queue out=w679:refnum<queue>, element=w678:string)  [unwired: 1 in, 2 out]
    n421 = Match Pattern(string=w678, regular expression=":") -> (before substring=w675:string, after substring=w676:string)  [unwired: 1 in, 2 out]
    n422 = case shown="\"init\"" w675 {
      tunnel: w679 -> [w692 w724 w757 w770 _ w858 w888 w953]
      tunnel: w676 -> [_ _ _ _ _ _ _ _]
      tunnel: [w686 w711 w756 w768 w811 w855 w873 w951] -> w674
      tunnel: w673 -> [_ _ w756 w768 w811 w855 w873 w951]
      tunnel: [w691 w725 u64 0 ("Hout") w767 w815 w856 w883 w950] -> w672
      tunnel: [w693 w726 w753 w766 w816 w857 w874 w949] -> w671
      tunnel: w670 -> [_ w728 w755 w767 w818 w860 w885 w950]
      tunnel: w669 -> [_ w727 _ w766 w817 w859 w884 w949]
      tunnel: [_ _ _ TRUE _ _ _ _] -> w668
      tunnel: [_ _ -1 _ _ _ _ -1] -> w666
      tunnel: [w685 w712 _ _ w825 _ _ _] -> w665
      tunnel: w664 -> [w685 w712 _ _ w824 _ _ _]
      tunnel: [w686 w714 w751 w765 w820 w849 w886 w948] -> w663
      tunnel: w662 -> [_ w714 w751 w765 w820 _ w886 w948]
      tunnel: w661 -> [_ _ _ _ _ _ w877 _]
      tunnel: [w683 w709 w750 w763 w778 w846 w880 w947] -> w660
      tunnel: w659 -> [w683 w709 w750 w763 w813 w846 w880 w947]
      tunnel: w658 -> [_ _ _ _ w786 _ _ _]
      tunnel: [w684 w710 w749 w764 w812 w845 w879 w946] -> w657
      tunnel: w656 -> [w684 w710 w749 w764 w785 w845 w879 w946]
      tunnel: [w682 w706 refnum<k21> refnum ("task out") w762 w771 w844 w870 w945] -> w655
      tunnel: w654 -> [_ w706 w748 w762 w771 w844 w871 w945]
      frame "init" {
        w686 = u16[][] []
        n423 = flat-sequence {
          tunnel: [w695] -> w690
          tunnel: [w696] -> w689
          tunnel: [w704] -> w691
          tunnel: [w705] -> w693
          tunnel: w690 -> [w705]
          tunnel: w689 -> [w704]
          frame #0 {
            n424 = local write "cam_con?"(FALSE ("cam_con?")) -> ()
          }
          frame #1 {
            n425 = call "SCInitBoard.vi"("boardnr"="board number") -> ("Hout"=w699:u32, "error out"=w700:errorcluster)  [unwired: 1 in, 1 out]
            n426 = call "SCSetupCamera.vi"("Handle"=w699, "error in (no error)"=w700) -> ("Hout"=w701:u64, "error out"=w702:errorcluster)  [unwired: 1 out]
            n427 = call "SCStopCOC.vi"("error in (no error)"=w702, "Stop mode"=0, "Handle"=w701) -> ("error out"=w695:errorcluster, "Hout"=w696:u64)
          }
          frame #2 {
            n428 = local write "cam_con?"(TRUE ("cam_con?")) -> ()
          }
        }
        n429 = Dequeue Element(queue=w692) -> (queue out=w688:refnum<queue>)  [unwired: 2 in, 3 out]
        n430 = Enqueue Element At Opposite End(queue=w688, element="set") -> ()  [unwired: 2 in, 3 out]
        n431 = call-poly <vilib>:"DAQmx Create Virtual Channel.vi"("lines"=tag "Dev2/port0/line7") -> ("task out"=w682:refnum<k21>)  [unwired: 13 in, 1 out]
      }
      frame "set" {
        n432 = Dequeue Element(queue=w724) -> ()  [unwired: 2 in, 4 out]
        n433 = call "SCStopCOC.vi"("error in (no error)"=w727, "Stop mode"=0, "Handle"=w728) -> ("error out"=w743:errorcluster, "Hout"=w742:u64)
        n434 = Bundle By Name(cluster=cluster{"Delay":dbl, "Exposure ":dbl} {"Delay"=0.0, "Exposure "=0.0} ("Delay and exposure"), "Exposure"="cam_exp") -> (w721:cluster{"Delay":dbl, "Exposure ":dbl})
        n435 = Bundle By Name(cluster=T10 {"Camera type"=0, "Operating mode\nHP & QE / HS & DiCam Pro "=0, "Frame trigger \n(High Performance and QE only)"=0, "Sequence trigger"=0, "Low Light\n(QE only)"=FALSE, "Gain"=FALSE, "Horzontal\nbinning"=0, "Vertical\nbinning "=0, "ROI Left"=1, "ROI Right"=20, "ROI Top"=1, "ROI Bottom"=15} ("Camera controls"), "Operating mode\nHP & QE / HS & DiCam Pro"="Operating mode\nHP & QE / HS & DiCam Pro", "Horzontal\nbinning"="binning", "Vertical\nbinning"="binning", "ROI Left"="ROI Left", "ROI Right"="ROI Right", "ROI Top"="ROI Top", "ROI Bottom"="ROI Bottom", "Gain"="gain", "Frame trigger \n(High Performance and QE only)"="Frame trigger \n(High Performance and QE only)") -> (w738:T10)
        n436 = call "New delay and exposure forma.vi"("Operating mode\nHP & QE / HS & DiCam Pro"="Operating mode\nHP & QE / HS & DiCam Pro", "Delay and exposure"=w721) -> ("Output table"=w739:string)  [unwired: 3 in]
        n437 = call "SCSetCoC.vi"("error in (no error)"=w743, "Delay and exposure table"=w739, "Camera controls"=w738, "Handle"=w742) -> ("error out"=w731:errorcluster, "Hout"=w730:u64)  [unwired: 1 out]
        n438 = call "SCGetImageSize.vi"("Handle"=w730, "error in (no error)"=w731) -> ("Hout"=w729:u64, "error out"=w713:errorcluster, "Horizontal size"=w718:i32, "Vertical size"=w717:i32)  [unwired: 2 out]
        n439 = Greater?(x=w718, y=w717) -> (0:w719:bool)
        n440 = Initialize Array(u16 0 ("dimension size"), w717, w718) -> (w711:u16[][])
        n441 = call "SCRun.vi"("error in (no error)"=w713, "Run mode"=0, "Handle"=w729) -> ("error out"=w726:errorcluster, "Hout"=w725:u64)  [unwired: 1 out]
        n442 = Select(t=w718, s=w719, f=w717) -> (s? t:f=w716:i32)
        n443 = property on="mainimg" class="IntGraph (strict)"("XScale.Maximum"=w716, "YScale.Maximum"=w716) -> ()  [unwired: 2 in, 2 out]
      }
      frame "release" {
        n444 = Dequeue Element(queue=w757) -> (queue out=w744:refnum<queue>)  [unwired: 2 in, 3 out]
        n445 = flat-sequence {
          tunnel: w755 -> [w759]
          tunnel: [w758] -> w752
          tunnel: [w761] -> w753
          tunnel: w752 -> [w761]
          frame #0 {
            n446 = call "SCCloseBoard.vi"("Handle"=w759) -> ("error out"=w758:errorcluster)  [unwired: 1 in, 2 out]
          }
          frame #1 {
            n447 = local write "cam_con?"(FALSE ("cam_con?")) -> ()
          }
        }
        n448 = Enqueue Element(queue=w744, element="suspend") -> ()  [unwired: 2 in, 3 out]
        n449 = call <vilib>:"DAQmx Clear Task.vi"("task in"=w748) -> ()  [unwired: 14 in, 1 out]
      }
      frame "close" {
        n450 = Release Queue(queue=w770) -> ()  [unwired: 2 in, 3 out]
      }
      frame "idle", Default {
        n451 = call "grabimg.vi"("array in"=w811, "error in"=w817, "Hin"=w818) -> ("error out"=w816:errorcluster, "imgdata"=w814:i32[][], "Hout"=w815:u64)  [unwired: 6 in]
        n452 = local read "lower threshold"() -> (w809:i32)
        n453 = case shown="False" "cam_dark?" {
          tunnel: w820 -> [_ w843]
          tunnel: [w840 w842] -> w810
          tunnel: w814 -> [w840 w841]
          frame False {
          }
          frame True {
            n454 = Subtract(x=w841, y=w843) -> (x-y=w842:dbl[][])
          }
        }
        n455 = call "filtr_b.vi"("threshold"=w809, "input array"=w810) -> ("output array"=w801:dbl[][])  [unwired: 9 in]
        n456 = call <vilib>:"High Resolution Relative Seconds.vi"() -> ("relative seconds"=w825:dbl)
        n457 = Subtract(x=w825, y=w824) -> (x-y=w823:dbl)
        n458 = Array Size(array=w801) -> (size(s)=w800:i32[])
        n459 = Reciprocal(x=w823) -> (1/x=→"cam_fps":dbl)
        n460 = Index Array(array=w800) -> (element #1=w795:i32, element #2=w794:i32)  [unwired: 2 in]
        n461 = Subtract(x=w786, y=w785) -> (x-y=w784:i32)
        n462 = Less Or Equal?(x="pics2avg", y=w784) -> (x <= y?=w807:bool)
        n463 = And(x="reset every n pics", y=w807) -> (x .and. y?=w805:bool)
        n464 = Not(x=w805) -> (.not. x?=w804:bool)
        n465 = call-poly <vilib>:"Ramp Pattern.vi"("start"=0.0, "end"=w795, "samples"=w795) -> ("Ramp Pattern"=w790:dbl[])  [unwired: 7 in, 1 out]
        n466 = call-poly <vilib>:"Ramp Pattern.vi"("start"=0.0, "end"=w794, "samples"=w794) -> ("Ramp Pattern"=w791:dbl[])  [unwired: 7 in, 1 out]
        n467 = property on="mainimg" class="IntGraph (strict)"() -> ("CrsrLis"=w783:T6)  [unwired: 2 in, 2 out]
        n468 = And(x="cam_liveavg", y=w804) -> (x .and. y?=w802:bool)
        n469 = case shown="False" w802 {
          tunnel: w801 -> [w830 w836]
          tunnel: [w830 w833] -> w778
          tunnel: w813 -> [_ w838]
          tunnel: w786 -> [w831 _]
          tunnel: [w831 w839] -> w812
          tunnel: w785 -> [_ w839]
          tunnel: w784 -> [_ w832]
          frame False {
          }
          frame True {
            n470 = Multiply(x=w838, y=w832) -> (x*y=w837:dbl[][])
            n471 = Increment(x=w832) -> (x+1=w834:i32)
            n472 = Add(x=w837, y=w836) -> (x+y=w835:dbl[][])
            n473 = Divide(x=w835, y=w834) -> (x/y=w833:dbl[][])
          }
        }
        "mainimg" <- w778
        n474 = Index Array(array=w783) -> (element #1=w781:T11, element #2=w782:T11)  [unwired: 2 in]
        n475 = Unbundle By Name(w781) -> ("Position.X"=w775:dbl, "Position.Y"=w777:dbl)
        n476 = Unbundle By Name(w782) -> ("Position.X"=w779:dbl, "Position.Y"=w780:dbl)
        n477 = Array Max & Min(array=w778) -> (max value=→"max":dbl)  [unwired: 3 out]
        n478 = Subtract(x=w780, y=w777) -> (x-y=w776:dbl)
        n479 = Subtract(x=w779, y=w775) -> (x-y=w774:dbl)
        n480 = Array Subset(array=w778, index (row)=w777, length (row)=w776) -> (w789:dbl[][])  [unwired: 2 in]
        n481 = Array Subset(array=w778, index (col)=w775, length (col)=w774) -> (w787:dbl[][])  [unwired: 2 in]
        n482 = Array Subset(array=w778, index (row)=w777, length (row)=w776, index (col)=w775, length (col)=w774) -> (w773:dbl[][])
        n483 = Transpose 2D Array(2D array=w789) -> (transposed array=w788:dbl[][])
        n484 = Add Array Elements(numeric array=w773) -> (sum=→"sum" →"Waveform Chart":dbl)
        n485 = for {
          tunnel: w787 -> [w827] mode=indexing
          tunnel: [w826] -> w797 mode=indexing
          n486 = Add Array Elements(numeric array=w827) -> (sum=w826:dbl)
        }
        n487 = for {
          tunnel: w788 -> [w829] mode=indexing
          tunnel: [w828] -> w796 mode=indexing
          n488 = Add Array Elements(numeric array=w829) -> (sum=w828:dbl)
        }
        n489 = Bundle("Ramp Pattern"=w791, w796) -> (→"G2 X":cluster{"Ramp Pattern":dbl[], dbl[]})  [unwired: 1 in]
        n490 = Bundle(w797, "Ramp Pattern"=w790) -> (→"G2 Y":cluster{dbl[], "Ramp Pattern":dbl[]})  [unwired: 1 in]
      }
      frame "dark" {
        n491 = Dequeue Element(queue=w858) -> ()  [unwired: 2 in, 4 out]
        n492 = Array Size(array=w855) -> (size(s)=w854:i32[])
        n493 = Index Array(array=w854) -> (element #1=w853:i32, element #2=w852:i32)  [unwired: 2 in]
        n494 = Initialize Array(0.0 ("element"), w853, w852) -> (w850:dbl[][])
        n495 = for {
          N: "dark avg" -> [_]
          tunnel: w860 -> [w868]
          tunnel: w859 -> [w867]
          tunnel: [w866] -> w857
          tunnel: w855 -> [w865]
          tunnel: [w864] -> w856
          shift-right: [w861] -> w848
          shift-left: w850 -> [w862]
          n496 = call "grabimg.vi"("array in"=w865, "error in"=w867, "Hin"=w868) -> ("error out"=w866:errorcluster, "imgdata"=w863:i32[][], "Hout"=w864:u64)  [unwired: 6 in]
          n497 = Add(x=w863, y=w862) -> (x+y=w861:dbl[][])
        }
        n498 = Divide(x=w848, y="dark avg") -> (x/y=w849:dbl[][])
      }
      frame "snap" {
        n499 = Dequeue Element(queue=w888) -> ()  [unwired: 2 in, 4 out]
        n500 = local read "cam_dark?"() -> (w887:bool)
        n501 = local read "cam_avgs"() -> (w882:i32)
        n502 = To Double Precision Float(number=w873) -> (double precision float=w872:dbl[][])
        n503 = Equal To 0?(x="aq.mode") -> (x = 0?=w875:bool)
        n504 = Get Date/Time In Seconds() -> (seconds since 1Jan1904=w878:timestamp)
        n505 = for {
          N: w882 -> [w900]
          shift-right: [w917] -> w883
          shift-left: w885 -> [w919]
          shift-right: [w905] -> w881
          shift-left: w884 -> [w918]
          tunnel: w887 -> [w915]
          tunnel: w886 -> [w914]
          tunnel: w873 -> [w913]
          tunnel: w878 -> [w909]
          tunnel: w875 -> [w893]
          shift-right: [w901] -> w869
          shift-left: w872 -> [w902]
          shift-right: [w891] -> w870
          shift-left: w871 -> [w891]
          i -> [w889]
          stop <- "abort acq." stop-if-true
          n506 = call "grabimg.vi"("array in"=w913, "error in"=w918, "Hin"=w919) -> ("error out"=w905:errorcluster, "imgdata"=w916:i32[][], "Hout"=w917:u64)  [unwired: 6 in]
          n507 = local read "lower threshold"() -> (w896:i32)
          n508 = Increment(x=w889) -> (x+1=w898:i32)
          "acq. imgs" <- w898
          n509 = Get Date/Time In Seconds() -> (seconds since 1Jan1904=w912:timestamp)
          n510 = case shown="True" w915 {
            tunnel: w916 -> [w941 w944]
            tunnel: w914 -> [_ w943]
            tunnel: [w941 w942] -> w895
            frame False {
            }
            frame True {
              n511 = Subtract(x=w944, y=w943) -> (x-y=w942:dbl[][])
            }
          }
          n512 = Divide(x=w898, y=w900) -> (x/y=→"snap_prog":dbl)
          n513 = Subtract(x=w912, y=w909) -> (x-y=w911:dbl)
          n514 = call "filtr_b.vi"("threshold"=w896, "input array"=w895) -> ("output array"=w894:dbl[][])  [unwired: 9 in]
          n515 = Divide(x=w911, y=w889) -> (x/y=w907:dbl)
          n516 = Multiply(x=w907, y=w900) -> (x*y=w910:dbl)
          n517 = Reciprocal(x=w907) -> (1/x=w906:dbl)
          n518 = case shown="True" "count?" {
            tunnel: w894 -> [w932 w934]
            tunnel: "e-size" -> [_ w936]
            tunnel: w896 -> [_ w935]
            tunnel: [w932 w933] -> w892
            frame False {
            }
            frame True {
              n519 = Array Size(array=w934) -> (size(s)=w938:i32[])
              n520 = call "findr.vi"("thresh"=w935, "esize"=w936, "inp array"=w934) -> ("locs"=w937:i32[][])  [unwired: 8 in]
              n521 = Index Array(array=w938) -> (element #1=w940:i32, element #2=w939:i32)  [unwired: 2 in]
              n522 = call "drawe.vi"("Ysize"=w940, "Xsize"=w939, "pos array"=w937) -> ("img out"=w933:i32[][])  [unwired: 8 in]
            }
          }
          n523 = Add(x=w910, y=w909) -> (x+y=→"ETA":timestamp)
          n524 = local write "cam_fps"(w906) -> ()
          n525 = local write "mainimg"(w894) -> ()
          n526 = case shown="True" w893 {
            tunnel: w892 -> [w922 w930]
            tunnel: w902 -> [w924 w929]
            tunnel: [w923 w927] -> w901
            tunnel: [w921 w926] -> w890
            tunnel: w889 -> [w920 w925]
            frame False {
              n527 = Add(x=w922, y=w924) -> (x+y=w923:dbl[][])
              n528 = Increment(x=w920) -> (x+1=w921:i32)
            }
            frame True {
              n529 = Multiply(x=w929, y=w925) -> (x*y=w931:dbl[][])
              n530 = Increment(x=w925) -> (x+1=w926:i32)
              n531 = Add(x=w930, y=w931) -> (x+y=w928:dbl[][])
              n532 = Divide(x=w928, y=w926) -> (x/y=w927:dbl[][])
            }
          }
          "Pics L" <- w890
          n533 = local write "sideimg"(w901) -> ()
        }
        n534 = Enqueue Element(queue=w877, element=w869, error in (no error)=w881) -> (error out=w874:errorcluster)  [unwired: 1 in, 2 out]
      }
      frame "suspend" {
        n535 = Dequeue Element(queue=w953) -> ()  [unwired: 2 in, 4 out]
      }
    }
    "cam_error" <- w671
  }
  n536 = while {
    tunnel: w10 -> [w962]
    shift-right: [w959] -> _
    shift-left: _ -> [w960]
    tunnel: w1 -> [w958]
    shift-right: [w957] -> _
    shift-left: _ -> [w956]
    shift-right: [w954] -> _
    shift-left: _ -> [w955]
    stop <- w961 stop-if-true
    # "mirr"
    n537 = Preview Queue Element(queue=w962, timeout in ms (-1)=w960) -> (queue out=w965:refnum<queue>, element=w966:string)  [unwired: 1 in, 2 out]
    n538 = Match Pattern(string=w966, regular expression=":") -> (before substring=w964:string, after substring=w963:string)  [unwired: 1 in, 2 out]
    n539 = case shown="\"abs\"" w964 {
      tunnel: w965 -> [w1001 w1011 w1026 w1030 w1033 w1038 _]
      tunnel: w963 -> [w995 w1012 _ _ _ _ _]
      tunnel: [_ _ _ TRUE _ _ _] -> w961
      tunnel: [_ _ _ _ -1 _ _] -> w959
      tunnel: w958 -> [w968 _ _ _ _ _ _]
      tunnel: [w987 w1008 refnum<visa-resource-name> refnum ("VISA resource name out") w1028 w1032 w1037 w1043] -> w957
      tunnel: w956 -> [w1000 w1010 w1025 w1028 w1032 _ w1047]
      tunnel: [w972 w1007 w1024 w1027 w1031 w1036 w1042] -> w954
      tunnel: w955 -> [w999 w1009 _ w1027 w1031 _ w1046]
      frame "abs" {
        w983 = u8 20 items=["Echo"=55, "Home"=1, "Move Absolute"=20, "Move Relative"=21, "Move at Constant Speed"=22, "Renumber"=2, "Restore Settings"=36, "Stop"=23] ("Command")
        w998 = u8 20 items=["Echo"=55, "Home"=1, "Move Absolute"=20, "Move Relative"=21, "Move at Constant Speed"=22, "Renumber"=2, "Restore Settings"=36, "Stop"=23] ("Command")
        n540 = Dequeue Element(queue=w1001) -> ()  [unwired: 2 in, 4 out]
        n541 = Match Pattern(string=w995, regular expression=":") -> (before substring=w985:string, after substring=w971:string)  [unwired: 1 in, 2 out]
        n542 = Equal?(x=w971, y="confirm") -> (x = y?=w969:bool)
        n543 = Scan From String(format string="%g_%g", input string=w985) -> (output 1=w980:dbl, output 2=w979:dbl)  [unwired: 4 in, 3 out]
        n544 = local read "mirr_X#"() -> (w982:u8)
        n545 = Bundle("mirr_X#"=w982, "Command"=w998, w980, "Response Count"=1) -> (w994:T12)  [unwired: 1 in]
        n546 = local read "mirr_Y#"() -> (w981:u8)
        n547 = call "Request Command.vi"("error in (no error)"=w999, "Request"=w994, "VISA resource name"=w1000) -> ("error out"=w976:errorcluster, "VISA resource name out"=w977:refnum<visa-resource-name>)  [unwired: 5 in, 2 out]
        n548 = Bundle("mirr_Y#"=w981, "Command"=w983, w979, "Response Count"=1) -> (w978:T13)  [unwired: 1 in]
        n549 = call "Request Command.vi"("error in (no error)"=w976, "Request"=w978, "VISA resource name"=w977) -> ("error out"=w974:errorcluster, "VISA resource name out"=w975:refnum<visa-resource-name>)  [unwired: 5 in, 2 out]
        n550 = local read "mirr_X#"() -> (w992:u8)
        n551 = call "zaber_readpos.vi"("error in (no error)"=w974, "axis"=w992, "VISA in"=w975) -> ("error out"=w988:errorcluster, "position"=w993:i32, "VISA out"=w989:refnum<visa-resource-name>)  [unwired: 6 in]
        n552 = local read "mirr_Y#"() -> (w990:u8)
        n553 = local write "mirr_posX"(w993) -> ()
        n554 = call "zaber_readpos.vi"("error in (no error)"=w988, "axis"=w990, "VISA in"=w989) -> ("error out"=w973:errorcluster, "position"=w991:i32, "VISA out"=w987:refnum<visa-resource-name>)  [unwired: 6 in]
        n555 = local write "mirr_posY"(w991) -> ()
        n556 = case shown="True" w969 {
          tunnel: w973 -> [w1002 w1006]
          tunnel: [w1002 w1005] -> w972
          tunnel: w968 -> [_ w1004]
          frame False {
          }
          frame True {
            n557 = Send Notification(notification=TRUE, notifier=w1004, error in (no error)=w1006) -> (error out=w1005:errorcluster)  [unwired: 1 out]
          }
        }
      }
      frame "rel" {
        w1015 = u8 21 items=["Echo"=55, "Home"=1, "Move Absolute"=20, "Move Relative"=21, "Move at Constant Speed"=22, "Renumber"=2, "Restore Settings"=36, "Stop"=23] ("Command")
        n558 = Dequeue Element(queue=w1011) -> ()  [unwired: 2 in, 4 out]
        n559 = Match Pattern(string=w1012, regular expression=":") -> (before substring=w1017:string, after substring=w1016:string)  [unwired: 1 in, 2 out]
        n560 = Decimal String To Number(string=w1017) -> (number=w1019:i32)  [unwired: 2 in, 1 out]
        n561 = Decimal String To Number(string=w1016) -> (number=w1020:i32)  [unwired: 2 in, 1 out]
        n562 = Bundle(w1019, "Command"=w1015, w1020, "Response Count"=1) -> (w1013:T14)  [unwired: 1 in]
        n563 = call "Request Command.vi"("error in (no error)"=w1009, "Request"=w1013, "VISA resource name"=w1010) -> ("error out"=w1007:errorcluster, "VISA resource name out"=w1008:refnum<visa-resource-name>)  [unwired: 5 in, 2 out]
      }
      frame "release" {
        n564 = Dequeue Element(queue=w1026) -> (queue out=w1022:refnum<queue>)  [unwired: 2 in, 3 out]
        n565 = Enqueue Element(queue=w1022, element="suspend") -> ()  [unwired: 2 in, 3 out]
        n566 = call "Close.vi"("VISA resource name"=w1025) -> ("error out"=w1024:errorcluster)  [unwired: 9 in, 1 out]
      }
      frame "close" {
        n567 = Release Queue(queue=w1030) -> ()  [unwired: 2 in, 3 out]
      }
      frame "suspend" {
        n568 = Dequeue Element(queue=w1033) -> ()  [unwired: 2 in, 4 out]
      }
      frame "init" {
        n569 = Dequeue Element(queue=w1038) -> ()  [unwired: 2 in, 4 out]
        n570 = call "Initialize.vi"("VISA resource name"="mirr_VISA") -> ("error out"=w1036:errorcluster, "VISA resource name out"=w1037:refnum<visa-resource-name>)  [unwired: 8 in, 1 out]
      }
      frame "idle", Default {
        n571 = local read "mirr_X#"() -> (w1048:u8)
        n572 = call "zaber_readpos.vi"("error in (no error)"=w1046, "axis"=w1048, "VISA in"=w1047) -> ("error out"=w1044:errorcluster, "position"=→"mirr_posX":i32, "VISA out"=w1045:refnum<visa-resource-name>)  [unwired: 6 in]
        n573 = local read "mirr_Y#"() -> (w1041:u8)
        n574 = call "zaber_readpos.vi"("error in (no error)"=w1044, "axis"=w1041, "VISA in"=w1045) -> ("error out"=w1042:errorcluster, "position"=→"mirr_posY":i32, "VISA out"=w1043:refnum<visa-resource-name>)  [unwired: 6 in]
      }
    }
    "mirr_Error" <- w954
  }
  n575 = while {
    tunnel: w18 -> [w1057]
    shift-right: [w1055] -> _
    shift-left: _ -> [w1053]
    shift-right: [w1054] -> _
    shift-left: _ -> [w1052]
    shift-right: [w1050] -> _
    shift-left: 0 -> [w1051]
    tunnel: w1 -> [w1049]
    stop <- w1056 stop-if-true
    # "ESP"
    n576 = Preview Queue Element(queue=w1057, timeout in ms (-1)=w1051) -> (queue out=w1060:refnum<queue>, element=w1061:string)  [unwired: 1 in, 2 out]
    n577 = Match Pattern(string=w1061, regular expression=":") -> (before substring=w1059:string, after substring=w1058:string)  [unwired: 1 in, 2 out]
    n578 = case shown="\"close\"" w1059 {
      tunnel: w1060 -> [_ w1072 w1090 w1131 w1134 w1141 w1146]
      tunnel: w1058 -> [_ w1077 w1097 _ _ _ _]
      tunnel: [_ _ _ _ _ TRUE _] -> w1056
      tunnel: [w1064 w1079 w1091 w1129 refnum<visa-resource-name> refnum ("VISA resource name out") w1138 w1145] -> w1055
      tunnel: [w1063 w1080 w1089 w1128 w1136 w1139 w1144] -> w1054
      tunnel: w1053 -> [w1068 w1082 w1095 w1129 w1137 w1138 _]
      tunnel: w1052 -> [w1067 w1081 w1096 w1128 _ w1139 _]
      tunnel: [_ _ _ -1 _ _ _] -> w1050
      tunnel: w1049 -> [_ _ w1083 _ _ _ _]
      frame "idle", Default {
        n579 = local read "ESP Axis"() -> (w1065:i32)
        n580 = local read "ESP_t0"() -> (w1071:dbl)
        n581 = call "Read Actual Position.vi"("error in (no error)"=w1067, "Axis (1)"=w1065, "VISA resource name"=w1068) -> ("error out"=w1063:errorcluster, "Position (units)"=w1066:dbl, "VISA resource name out"=w1064:refnum<visa-resource-name>)  [unwired: 2 in]
        "ESP_pos" <- w1066
        n582 = call "mm2time.vi"("fs?"=TRUE, "Offset (mm)"=w1071, "distance (mm)"=w1066) -> ("time in fs/ps seconds"=→"ESP_delay":dbl)
      }
      frame "rel" {
        n583 = Match Pattern(string=w1077, regular expression=":") -> (before substring=w1076:string, after substring=w1075:string)  [unwired: 1 in, 2 out]
        n584 = Dequeue Element(queue=w1072) -> ()  [unwired: 2 in, 4 out]
        n585 = Decimal String To Number(string=w1076) -> (number=w1074:i32)  [unwired: 2 in, 1 out]
        n586 = Fract/Exp String To Number(string=w1075) -> (number=w1073:dbl)  [unwired: 3 in, 1 out]
        n587 = call "Move Relative.vi"("error in (no error)"=w1081, "Position (0 units)"=w1073, "Axis (1)"=w1074, "VISA resource name"=w1082) -> ("error out"=w1080:errorcluster, "VISA resource name out"=w1079:refnum<visa-resource-name>)  [unwired: 2 in]
      }
      frame "abs" {
        n588 = Dequeue Element(queue=w1090) -> ()  [unwired: 2 in, 4 out]
        n589 = Match Pattern(string=w1097, regular expression=":") -> (before substring=w1098:string, after substring=w1087:string)  [unwired: 1 in, 2 out]
        n590 = Match Pattern(string=w1087, regular expression=":") -> (before substring=w1086:string, after substring=w1085:string)  [unwired: 1 in, 2 out]
        n591 = Decimal String To Number(string=w1098) -> (number=w1094:i32)  [unwired: 2 in, 1 out]
        n592 = Fract/Exp String To Number(string=w1086) -> (number=w1084:dbl)  [unwired: 3 in, 1 out]
        n593 = call "Move Absolute.vi"("error in (no error)"=w1096, "Position (0 units)"=w1084, "Axis (1)"=w1094, "VISA resource name"=w1095) -> ("error out"=w1092:errorcluster, "VISA resource name out"=w1093:refnum<visa-resource-name>)  [unwired: 2 in]
        n594 = case shown="\"confirm\"" w1085 {
          tunnel: w1094 -> [_ w1116]
          tunnel: w1093 -> [w1101 w1118]
          tunnel: w1092 -> [w1100 w1117]
          tunnel: [w1101 w1104] -> w1091
          tunnel: [w1100 w1113] -> w1089
          tunnel: w1083 -> [_ w1112]
          frame "", Default {
          }
          frame "confirm" {
            n595 = while {
              tunnel: w1116 -> [w1127]
              shift-right: [w1124] -> w1115
              shift-left: w1118 -> [w1126]
              shift-right: [w1123] -> w1114
              shift-left: w1117 -> [w1125]
              stop <- w1122 stop-if-true
              n596 = call "Get Axis Motion Status.vi"("error in (no error)"=w1125, "Axis (1)"=w1127, "VISA resource name"=w1126) -> ("error out"=w1123:errorcluster, "Motion Done"=w1122:bool, "VISA resource name out"=w1124:refnum<visa-resource-name>)  [unwired: 2 in]
            }
            n597 = flat-sequence {
              tunnel: w1115 -> [w1121]
              tunnel: w1114 -> [w1120]
              tunnel: [w1121] -> w1107
              tunnel: [w1120] -> w1106
              frame #0 {
                n598 = Wait (ms)(milliseconds to wait=u32 1000) -> ()  [unwired: 1 out]
              }
            }
            n599 = local read "ESP Axis"() -> (w1108:i32)
            n600 = local read "ESP_t0"() -> (w1110:dbl)
            n601 = call "Read Actual Position.vi"("error in (no error)"=w1106, "Axis (1)"=w1108, "VISA resource name"=w1107) -> ("error out"=w1105:errorcluster, "Position (units)"=w1102:dbl, "VISA resource name out"=w1104:refnum<visa-resource-name>)  [unwired: 2 in]
            n602 = call "mm2time.vi"("fs?"=TRUE, "Offset (mm)"=w1110, "distance (mm)"=w1102) -> ("time in fs/ps seconds"=w1103:dbl)
            n603 = local write "ESP_pos"(w1102) -> ()
            n604 = local write "ESP_delay"(w1103) -> ()
            n605 = Send Notification(notification=TRUE, notifier=w1112, error in (no error)=w1105) -> (error out=w1113:errorcluster)  [unwired: 1 out]
          }
        }
      }
      frame "suspend" {
        n606 = Dequeue Element(queue=w1131) -> ()  [unwired: 2 in, 4 out]
      }
      frame "release" {
        n607 = Dequeue Element(queue=w1134) -> (queue out=w1132:refnum<queue>)  [unwired: 2 in, 3 out]
        n608 = call "Close.vi"("VISA resource name"=w1137) -> ("error out"=w1136:errorcluster)  [unwired: 10 in]
        n609 = Enqueue Element(queue=w1132, element="suspend") -> ()  [unwired: 2 in, 3 out]
      }
      frame "close" {
        n610 = Release Queue(queue=w1141) -> ()  [unwired: 2 in, 3 out]
      }
      frame "init" {
        n611 = Dequeue Element(queue=w1146) -> ()  [unwired: 2 in, 4 out]
        n612 = flat-sequence {
          tunnel: [w1149] -> w1143
          tunnel: [w1148] -> w1142
          tunnel: [w1153] -> w1144
          tunnel: [w1154] -> w1145
          tunnel: w1143 -> [w1154]
          tunnel: w1142 -> [w1153]
          frame #0 {
            n613 = local write "ESP_con?"(FALSE ("ESP_con?")) -> ()
          }
          frame #1 {
            n614 = call "Initialize.vi"("VISA resource name"="ESP301 VISA", "Serial Link (RS232)"=enum16{"RS232", "USB"}."USB") -> ("VISA resource name out"=w1149:refnum<visa-resource-name>, "error out"=w1148:errorcluster)  [unwired: 7 in]
          }
          frame #2 {
            n615 = local write "ESP_con?"(TRUE ("ESP_con?")) -> ()
          }
        }
      }
    }
    "error out" <- w1054
  }
  n616 = while {
    tunnel: w17 -> [w1163]
    shift-right: [w1161] -> _
    shift-left: _ -> [w1159]
    shift-right: [w1160] -> _
    shift-left: _ -> [w1158]
    shift-right: [w1156] -> _
    shift-left: 0 -> [w1157]
    tunnel: w1 -> [w1155]
    stop <- w1162 stop-if-true
    # "manip"
    n617 = Preview Queue Element(queue=w1163, timeout in ms (-1)=w1157) -> (queue out=w1166:refnum<queue>, element=w1167:string)  [unwired: 1 in, 2 out]
    n618 = Match Pattern(string=w1167, regular expression=":") -> (before substring=w1165:string, after substring=w1164:string)  [unwired: 1 in, 2 out]
    n619 = case shown="\"rel\"" w1165 {
      tunnel: w1166 -> [_ w1179 w1206 w1253 w1291 w1297 w1306 w1311]
      tunnel: w1164 -> [_ _ w1193 w1252 _ _ _ _]
      tunnel: [_ _ _ _ _ _ TRUE _] -> w1162
      tunnel: [w1173 w1181 w1185 w1250 w1293 refnum<k5> refnum ("gateway_connection out") w1304 w1310] -> w1161
      tunnel: [w1172 w1180 w1187 w1249 w1292 w1299 w1303 w1309] -> w1160
      tunnel: w1159 -> [w1175 w1183 w1209 w1243 w1293 w1301 w1304 _]
      tunnel: w1158 -> [w1174 w1182 w1208 w1244 w1292 _ w1303 _]
      tunnel: [_ _ _ _ -1 _ _ _] -> w1156
      tunnel: w1155 -> [_ _ w1184 w1246 _ _ _ _]
      frame "idle", Default {
        n620 = call "sp_manip_get_axis_status.vi"("error in"=w1174, "gateway_connection"=w1175) -> ("error out"=w1172:errorcluster, "axis_out"=w1171:T15, "gateway_connection out"=w1173:refnum<k5>)  [unwired: 5 in, 2 out]
        n621 = for {
          tunnel: w1171 -> [w1178] mode=indexing
          tunnel: [w1177] -> w1170 mode=indexing
          tunnel: [w1176] -> w1169 mode=indexing
          n622 = Unbundle By Name(w1178) -> ("Axis_Position"=w1177:dbl, "moving"=w1176:bool)
        }
        "moving?" <- w1169
        n623 = local write "pos"(w1170) -> ()
      }
      frame "stop" {
        n624 = Dequeue Element(queue=w1179) -> ()  [unwired: 2 in, 4 out]
        n625 = call "sp_manip_abort.vi"("error in"=w1182, "gateway_connection"=w1183) -> ("error out"=w1180:errorcluster, "gateway_connection out"=w1181:refnum<k5>)  [unwired: 6 in, 2 out]
      }
      frame "rel" {
        n626 = Dequeue Element(queue=w1206) -> ()  [unwired: 2 in, 4 out]
        n627 = Match Pattern(string=w1193, regular expression=":") -> (before substring=w1192:string, after substring=w1191:string)  [unwired: 1 in, 2 out]
        n628 = Equal?(x=w1191, y="confirm") -> (x = y?=w1189:bool)
        n629 = call "sp_manip_get_axis_status.vi"("error in"=w1208, "gateway_connection"=w1209) -> ("error out"=w1211:errorcluster, "axis_out"=w1198:T15, "gateway_connection out"=w1210:refnum<k5>)  [unwired: 5 in, 2 out]
        n630 = Scan From String(format string="%g_%g_%g_%g_%g_%g", input string=w1192) -> (output 1=w1205:dbl, output 2=w1204:dbl, output 3=w1203:dbl, output 4=w1202:dbl, output 5=w1201:dbl, output 6=w1200:dbl)  [unwired: 8 in, 3 out]
        n631 = for {
          tunnel: w1198 -> [w1238] mode=indexing
          tunnel: [w1237] -> w1196 mode=indexing
          tunnel: [w1236] -> w1197 mode=indexing
          n632 = Unbundle By Name(w1238) -> ("Axis_Name"=w1237:string, "Axis_Position"=w1236:dbl)
        }
        n633 = Build Array(w1205, w1204, w1203, w1202, w1201, w1200) -> (w1199:dbl[])
        n634 = Add(x=w1197, y=w1199) -> (x+y=w1195:dbl[])
        n635 = call "sp_manip_start_move.vi"("error in"=w1211, "target positions"=w1195, "axis names"=w1196, "gateway_connection"=w1210) -> ("error out"=w1188:errorcluster, "gateway_connection out"=w1186:refnum<k5>)  [unwired: 4 in, 2 out]
        n636 = case shown="True" w1189 {
          tunnel: w1188 -> [w1212 w1223]
          tunnel: [w1212 w1222] -> w1187
          tunnel: w1186 -> [w1213 w1224]
          tunnel: [w1213 w1215] -> w1185
          tunnel: w1184 -> [_ w1221]
          frame False {
          }
          frame True {
            n637 = while {
              tunnel: w1224 -> [w1230]
              tunnel: w1223 -> [w1229]
              tunnel: [w1228] -> w1216
              tunnel: [w1227] -> w1218
              stop <- w1231 continue-if-true
              n638 = call "sp_manip_get_axis_status.vi"("error in"=w1229, "gateway_connection"=w1230) -> ("error out"=w1227:errorcluster, "axis_out"=w1233:T15, "gateway_connection out"=w1228:refnum<k5>)  [unwired: 5 in, 2 out]
              n639 = for {
                tunnel: w1233 -> [w1235] mode=indexing
                tunnel: [w1234] -> w1232 mode=indexing
                n640 = Unbundle By Name(w1235) -> ("moving"=w1234:bool)
              }
              n641 = Or Array Elements(Boolean array=w1232) -> (logical OR=w1231:bool)
            }
            n642 = call "sp_manip_get_axis_status.vi"("error in"=w1218, "gateway_connection"=w1216) -> ("error out"=w1217:errorcluster, "axis_out"=w1219:T15, "gateway_connection out"=w1215:refnum<k5>)  [unwired: 5 in, 2 out]
            n643 = for {
              tunnel: w1219 -> [w1226] mode=indexing
              tunnel: [w1225] -> w1214 mode=indexing
              n644 = Unbundle By Name(w1226) -> ("Axis_Position"=w1225:dbl)
            }
            n645 = Send Notification(notification=TRUE, notifier=w1221, error in (no error)=w1217) -> (error out=w1222:errorcluster)  [unwired: 1 out]
            n646 = local write "dest"(w1214) -> ()
          }
        }
      }
      frame "abs" {
        n647 = Dequeue Element(queue=w1253) -> ()  [unwired: 2 in, 4 out]
        n648 = call "sp_manip_get_axis_status.vi"("error in"=w1244, "gateway_connection"=w1243) -> ("error out"=w1239:errorcluster, "axis_out"=w1242:T15, "gateway_connection out"=w1240:refnum<k5>)  [unwired: 5 in, 2 out]
        n649 = Match Pattern(string=w1252, regular expression=":") -> (before substring=w1256:string, after substring=w1255:string)  [unwired: 1 in, 2 out]
        n650 = Equal?(x=w1255, y="wait") -> (x = y?=w1245:bool)
        n651 = for {
          tunnel: w1242 -> [w1266] mode=indexing
          tunnel: [w1265] -> w1241 mode=indexing
          n652 = Unbundle By Name(w1266) -> ("Axis_Name"=w1265:string)
        }
        n653 = Scan From String(format string="%g_%g_%g_%g_%g_%g", input string=w1256) -> (output 1=w1262:dbl, output 2=w1261:dbl, output 3=w1260:dbl, output 4=w1259:dbl, output 5=w1258:dbl, output 6=w1257:dbl)  [unwired: 8 in, 3 out]
        n654 = Build Array(w1262, w1261, w1260, w1259, w1258, w1257) -> (w1264:dbl[])
        n655 = call "sp_manip_start_move.vi"("error in"=w1239, "target positions"=w1264, "axis names"=w1241, "gateway_connection"=w1240) -> ("error out"=w1248:errorcluster, "gateway_connection out"=w1247:refnum<k5>)  [unwired: 4 in, 2 out]
        n656 = case shown="True" w1245 {
          tunnel: w1248 -> [w1267 w1278]
          tunnel: [w1267 w1277] -> w1249
          tunnel: w1247 -> [w1268 w1279]
          tunnel: [w1268 w1270] -> w1250
          tunnel: w1246 -> [_ w1276]
          frame False {
          }
          frame True {
            n657 = while {
              tunnel: w1279 -> [w1285]
              tunnel: w1278 -> [w1284]
              tunnel: [w1283] -> w1272
              tunnel: [w1282] -> w1271
              stop <- w1286 continue-if-true
              n658 = call "sp_manip_get_axis_status.vi"("error in"=w1284, "gateway_connection"=w1285) -> ("error out"=w1282:errorcluster, "axis_out"=w1288:T15, "gateway_connection out"=w1283:refnum<k5>)  [unwired: 5 in, 2 out]
              n659 = for {
                tunnel: w1288 -> [w1290] mode=indexing
                tunnel: [w1289] -> w1287 mode=indexing
                n660 = Unbundle By Name(w1290) -> ("moving"=w1289:bool)
              }
              n661 = Or Array Elements(Boolean array=w1287) -> (logical OR=w1286:bool)
            }
            n662 = call "sp_manip_get_axis_status.vi"("error in"=w1271, "gateway_connection"=w1272) -> ("error out"=w1269:errorcluster, "axis_out"=w1274:T15, "gateway_connection out"=w1270:refnum<k5>)  [unwired: 5 in, 2 out]
            n663 = for {
              tunnel: w1274 -> [w1281] mode=indexing
              tunnel: [w1280] -> w1273 mode=indexing
              n664 = Unbundle By Name(w1281) -> ("Axis_Position"=w1280:dbl)
            }
            n665 = local write "pos"(w1273) -> ()
            n666 = Send Notification(notification=TRUE, notifier=w1276, error in (no error)=w1269) -> (error out=w1277:errorcluster)  [unwired: 1 out]
          }
        }
      }
      frame "suspend" {
        n667 = Dequeue Element(queue=w1291) -> ()  [unwired: 2 in, 4 out]
      }
      frame "release" {
        n668 = Dequeue Element(queue=w1297) -> (queue out=w1295:refnum<queue>)  [unwired: 2 in, 3 out]
        n669 = call "sp_manip_disconnect.vi"("gateway_connection"=w1301) -> ("error out"=w1300:errorcluster, "gateway_connection_out"=w1302:refnum<k5>)  [unwired: 7 in, 2 out]
        n670 = call "tcp_gateway_close_connection.vi"("error in"=w1300, "server_connection"=w1302) -> ("error out"=w1299:errorcluster)  [unwired: 5 in]
        n671 = Enqueue Element(queue=w1295, element="suspend") -> ()  [unwired: 2 in, 3 out]
      }
      frame "close" {
        n672 = Release Queue(queue=w1306) -> ()  [unwired: 2 in, 3 out]
      }
      frame "init" {
        n673 = Dequeue Element(queue=w1311) -> ()  [unwired: 2 in, 4 out]
        n674 = flat-sequence {
          tunnel: [w1314] -> w1308
          tunnel: [w1313] -> w1307
          tunnel: [w1324] -> w1309
          tunnel: [w1325] -> w1310
          tunnel: w1308 -> [w1325]
          tunnel: w1307 -> [w1324]
          frame #0 {
            n675 = local write "manip_con?"(FALSE ("manip_con?")) -> ()
          }
          frame #1 {
            n676 = call "tcp_gateway_open_connection.vi"() -> ("gateway_connection"=w1317:refnum<k5>, "error out"=w1316:errorcluster)  [unwired: 5 in, 3 out]
            n677 = call "sp_manip_connect.vi"("error in"=w1316, "gateway_connection"=w1317) -> ("error out"=w1313:errorcluster, "axis_out"=w1315:T15, "gateway_connection out"=w1314:refnum<k5>)  [unwired: 5 in, 2 out]
            n678 = for {
              tunnel: w1315 -> [w1322] mode=indexing
              tunnel: [w1321] -> w1318 mode=indexing
              tunnel: [w1320] -> w1319 mode=indexing
              n679 = Unbundle By Name(w1322) -> ("Axis_Name"=w1321:string, "Axis_Position"=w1320:dbl)
            }
            "axis" <- w1318
            "pos" <- w1319
            n680 = local write "dest"(w1319) -> ()
          }
          frame #2 {
            n681 = local write "manip_con?"(TRUE ("manip_con?")) -> ()
          }
        }
      }
    }
    "error out 2" <- w1160
  }
  n682 = while {
    tunnel: w16 -> [w1337]
    shift-right: [w1326] -> _
    shift-left: 0 -> [w1335]
    shift-right: [w1334] -> _
    shift-left: _ -> [w1333]
    shift-right: [w1332] -> _
    shift-left: _ -> [w1331]
    shift-right: [w1330] -> _
    shift-left: u32 0 ("pHandle") -> [w1329]
    tunnel: w15 -> [w1328]
    tunnel: w1 -> [w1327]
    stop <- w1336 stop-if-true
    # "phoib"
    n683 = Preview Queue Element(queue=w1337, timeout in ms (-1)=w1335) -> (queue out=w1340:refnum<queue>, element=w1341:string)  [unwired: 1 in, 2 out]
    n684 = Match Pattern(string=w1341, regular expression=":") -> (before substring=w1339:string, after substring=w1338:string)  [unwired: 1 in, 2 out]
    n685 = case shown="\"idle\", Default" w1339 {
      tunnel: w1340 -> [_ w1394 w1448 w1465 w1483 w1497 w1502 w1507]
      tunnel: w1338 -> [_ _ w1444 _ _ _ _ _]
      tunnel: [_ _ _ _ _ TRUE _ _] -> w1336
      tunnel: [w1351 w1396 w1413 w1468 w1481 w1495 w1501 w1504] -> w1334
      tunnel: w1333 -> [w1362 w1385 w1434 w1470 w1482 w1495 w1501 _]
      tunnel: [w1350 w1395 w1429 w1467 w1480 w1493 w1499 w1503] -> w1332
      tunnel: w1331 -> [w1360 w1384 _ w1469 _ w1493 w1499 _]
      tunnel: [w1348 w1382 w1412 w1466 w1479 w1494 w1500 w1506] -> w1330
      tunnel: w1329 -> [w1348 w1382 w1432 w1466 w1478 w1494 w1500 _]
      tunnel: w1328 -> [w1349 w1375 w1410 _ _ _ _ _]
      tunnel: w1327 -> [_ _ w1428 _ _ _ _ _]
      tunnel: [_ _ _ _ _ _ -1 _] -> w1326
      frame "idle", Default {
        n686 = call "SL2_AD_DLL_Phoibos_GetDeviceState.vi"("dll_path"=w1362, "pHandle_in"=w1348, "dev_type"=DEF_dev_type."devA (analyzer)", "error in"=w1360) -> ("path out"=w1347:path, "state"=→"state":T4, "error out"=w1346:errorcluster)  [unwired: 2 in]
        n687 = for {
          tunnel: w1348 -> [w1369]
          tunnel: w1349 -> [w1367] mode=indexing
          tunnel: [w1366] -> w1359 mode=indexing
          tunnel: [w1365] -> w1351
          shift-right: [w1364] -> w1350
          shift-left: w1346 -> [w1368]
          tunnel: w1347 -> [w1363]
          n688 = call "SL2_AD_DLL_Phoibos_GetVoltage.vi"("error in"=w1368, "voltage_name"=w1367, "pHandle"=w1369, "dll path in"=w1363) -> ("error out"=w1364:errorcluster, "value"=w1366:dbl, "dll path out"=w1365:path)  [unwired: 3 in]
        }
        n689 = Index Array(array=w1359) -> (element #1=→"phoib_I_1":dbl, element #2=→"phoib_I_2":dbl, element #3=→"phoib_I_3":dbl, element #4=→"phoib_I_4":dbl, element #5=→"phoib_I_5":dbl, element #6=→"phoib_I_6":dbl, element #7=→"phoib_I_7":dbl, element #8=→"phoib_I_8":dbl, element #9=→"phoib_I_9":dbl)  [unwired: 9 in]
      }
      frame "set" {
        n690 = Dequeue Element(queue=w1394) -> ()  [unwired: 2 in, 4 out]
        n691 = Multiply(x="ana_voltrange", y=13) -> (x*y=w1391:i32)
        n692 = Add(x="ana_mode", y=w1391) -> (x+y=w1388:i32)
        n693 = Index Array(array=u32[] [251749632, 251749633, 251749634, 251749635, 251749636, 251749637, 251749638, 251749639, 251749640, 251749641, 251749642, 251749643, 251749644, 251749645, 251749646, 251749647, 251749648, 251749649, 251749650, 251749651, 251749652, 251749653, 251749654, 251749655, 251749656, 251749657, 251749658, 251749659, 251749660, 251749661, 251749662, 251749663, 251749664, 251749665, 251749666, 251749667, 251749668, 251749669, 251749670, 251749671, 251749672, 251749673, 251749674, 251749675, 251749676, 251749677, 251749678, 251749679, 251749680, 251749681, 251749682, 251749683, 251749684, 251749685, 251749686, 251749687, 251749688, 251749689, 251749690, 251749691, 251749692, 251749693, 251749694, 251749695, 251749696] ("modeIDs"), index=w1388) -> (element=w1386:u32)
        n694 = Build Array("phoib_I_1s", "phoib_I_2s", "phoib_I_3s", "phoib_I_4s", "phoib_I_5s", "phoib_I_6s", "phoib_I_7s", "phoib_I_8s", "phoib_I_9s") -> (w1374:dbl[])
        n695 = call "SL2_AD_DLL_Phoibos_SetDeviceMode.vi"("pHandle"=w1382, "error in"=w1384, "value"=w1386, "dev_type"=DEF_dev_type."devA (analyzer)", "dll path in"=w1385) -> ("error out"=w1373:errorcluster, "dll path out"=w1383:path)  [unwired: 4 in]
        n696 = for {
          tunnel: w1382 -> [w1402]
          shift-right: [w1409] -> w1396
          shift-left: w1383 -> [w1406]
          tunnel: w1375 -> [w1401] mode=indexing
          tunnel: w1374 -> [w1400] mode=indexing
          shift-right: [w1408] -> w1395
          shift-left: w1373 -> [w1404]
          n697 = call "SL2_AD_DLL_Phoibos_GetVoltageRange.vi"("error in"=w1404, "voltage_name"=w1401, "pHandle"=w1402, "dll path in"=w1406) -> ("error out"=w1403:errorcluster, "min"=w1398:dbl, "max"=w1399:dbl, "dll path out"=w1405:path)  [unwired: 2 in]
          n698 = In Range and Coerce(upper limit=w1399, x=w1400, lower limit=w1398) -> (coerced(x)=w1397:dbl)  [unwired: 1 out]
          n699 = call "SL2_AD_DLL_Phoibos_SetVoltage.vi"("commit"=TRUE, "pHandle"=w1402, "error in"=w1403, "value"=w1397, "voltageName"=w1401, "dll path in"=w1405) -> ("error out"=w1408:errorcluster, "dll path out"=w1409:path)  [unwired: 3 in]
        }
      }
      frame "setsgl" {
        n700 = Dequeue Element(queue=w1448) -> ()  [unwired: 2 in, 4 out]
        n701 = Match Pattern(string=w1444, regular expression=":") -> (before substring=w1437:string, after substring=w1446:string)  [unwired: 1 in, 2 out]
        n702 = Equal?(x=w1446, y="wait") -> ()  [unwired: 1 out]
        n703 = Match Pattern(string=w1437, regular expression=":") -> (before substring=w1411:string, after substring=w1436:string)  [unwired: 1 in, 2 out]
        n704 = Fract/Exp String To Number(string=w1436) -> (number=w1435:dbl)  [unwired: 3 in, 1 out]
        n705 = call "SL2_AD_DLL_Phoibos_GetVoltageRange.vi"("voltage_name"=w1411, "pHandle"=w1432, "dll path in"=w1434) -> ("error out"=w1441:errorcluster, "min"=w1439:dbl, "max"=w1440:dbl, "dll path out"=w1442:path)  [unwired: 3 in]
        n706 = In Range and Coerce(upper limit=w1440, x=w1435, lower limit=w1439) -> (coerced(x)=w1430:dbl)  [unwired: 1 out]
        n707 = call "SL2_AD_DLL_Phoibos_SetVoltage.vi"("commit"=TRUE, "pHandle"=w1432, "error in"=w1441, "value"=w1430, "voltageName"=w1411, "dll path in"=w1442) -> ("error out"=w1431:errorcluster, "dll path out"=w1433:path)  [unwired: 3 in]
        n708 = while {
          tunnel: w1433 -> [w1464]
          tunnel: w1432 -> [w1458]
          tunnel: w1411 -> [w1463]
          tunnel: w1431 -> [w1462]
          tunnel: w1430 -> [w1461]
          tunnel: [w1458] -> w1412
          tunnel: [w1457] -> w1414
          tunnel: [w1456] -> w1416
          stop <- w1459 stop-if-true
          n709 = call "SL2_AD_DLL_Phoibos_GetVoltage.vi"("error in"=w1462, "voltage_name"=w1463, "pHandle"=w1458, "dll path in"=w1464) -> ("error out"=w1456:errorcluster, "value"=w1460:dbl, "dll path out"=w1457:path)  [unwired: 3 in]
          n710 = Equal?(x=w1461, y=w1460) -> (x = y?=w1459:bool)
        }
        n711 = for {
          tunnel: w1412 -> [w1455]
          tunnel: [w1453] -> w1417 mode=indexing
          tunnel: [w1452] -> w1413
          shift-right: [w1451] -> w1415
          shift-left: w1416 -> [w1454]
          tunnel: w1414 -> [w1450]
          tunnel: w1410 -> [w1449] mode=indexing
          n712 = call "SL2_AD_DLL_Phoibos_GetVoltage.vi"("error in"=w1454, "voltage_name"=w1449, "pHandle"=w1455, "dll path in"=w1450) -> ("error out"=w1451:errorcluster, "value"=w1453:dbl, "dll path out"=w1452:path)  [unwired: 3 in]
        }
        n713 = Index Array(array=w1417) -> (element #1=w1418:dbl, element #2=w1419:dbl, element #3=w1420:dbl, element #4=w1421:dbl, element #5=w1422:dbl, element #6=w1426:dbl, element #7=w1423:dbl, element #8=w1424:dbl, element #9=w1425:dbl)  [unwired: 9 in]
        n714 = local write "phoib_I_1"(w1418) -> ()
        n715 = local write "phoib_I_2"(w1419) -> ()
        n716 = local write "phoib_I_3"(w1420) -> ()
        n717 = local write "phoib_I_4"(w1421) -> ()
        n718 = local write "phoib_I_5"(w1422) -> ()
        n719 = local write "phoib_I_6"(w1426) -> ()
        n720 = local write "phoib_I_7"(w1423) -> ()
        n721 = local write "phoib_I_8"(w1424) -> ()
        n722 = local write "phoib_I_9"(w1425) -> ()
        n723 = Send Notification(notification=TRUE, notifier=w1428, error in (no error)=w1415) -> (error out=w1429:errorcluster)  [unwired: 1 out]
      }
      frame "standby" {
        w1471 = T4 0 items=["Off"=-1, "Standby"=0, "On"=1] ("state")
        n724 = Dequeue Element(queue=w1465) -> ()  [unwired: 2 in, 4 out]
        n725 = call "SL2_AD_DLL_Phoibos_SetDeviceState.vi"("pHandle_in"=w1466, "error in"=w1469, "state"=w1471, "dev_type"=DEF_dev_type."devA (analyzer)", "dll_path"=w1470) -> ("error out"=w1467:errorcluster, "path out"=w1468:path)  [unwired: 2 in]
      }
      frame "release" {
        n726 = Dequeue Element(queue=w1483) -> (queue out=w1473:refnum<queue>)  [unwired: 2 in, 3 out]
        n727 = flat-sequence {
          tunnel: w1482 -> [w1484]
          tunnel: w1478 -> [w1485]
          tunnel: [w1488] -> w1477
          tunnel: [w1487] -> w1476
          tunnel: [u32 0] -> w1475
          tunnel: [w1490] -> w1479
          tunnel: [w1491] -> w1480
          tunnel: [w1492] -> w1481
          tunnel: w1477 -> [w1492]
          tunnel: w1476 -> [w1491]
          tunnel: w1475 -> [w1490]
          frame #0 {
            n728 = call "SL2_AD_DLL_Phoibos_Shutdown.vi"("pHandle"=w1485, "dll path in"=w1484) -> ("error out"=w1487:errorcluster, "dll path out"=w1488:path)  [unwired: 4 in]
          }
          frame #1 {
            n729 = local write "phoib_con?"(FALSE ("phoib_con?")) -> ()
          }
        }
        n730 = Enqueue Element(queue=w1473, element="suspend") -> ()  [unwired: 2 in, 3 out]
      }
      frame "close" {
        n731 = Release Queue(queue=w1497) -> ()  [unwired: 2 in, 3 out]
      }
      frame "suspend" {
        n732 = Dequeue Element(queue=w1502) -> ()  [unwired: 2 in, 4 out]
      }
      frame "init" {
        n733 = Dequeue Element(queue=w1507) -> ()  [unwired: 2 in, 4 out]
        n734 = flat-sequence {
          tunnel: [w1514] -> w1505
          tunnel: [w1510] -> w1504
          tunnel: [w1509] -> w1503
          tunnel: [w1522] -> w1506
          tunnel: w1505 -> [w1522]
          frame #0 {
            n735 = local write "phoib_con?"(FALSE ("phoib_con?")) -> ()
          }
          frame #1 {
            w1513 = DEF_dev_type."devA (analyzer)" ("dev_type")
            n736 = call "GetSL2AD_VI_dllPath.vi"() -> ("error"=w1517:errorcluster, "Path"=w1518:path)  [unwired: 9 in, 1 out]
            n737 = call "SL2_AD_DLL_List_Devices.vi"("error in"=w1517, "dev_type"=w1513, "dll path in"=w1518) -> ("error out"=w1511:errorcluster, "devices"=w1520:string[], "dll path out"=w1512:path)  [unwired: 2 in]
            n738 = Index Array(array=w1520) -> (element=w1519:string)  [unwired: 1 in]
            n739 = call "SL2_AD_DLL_Phoibos_Initialize.vi"("error in"=w1511, "analyzerId"=w1519, "dll_path"=w1512) -> ("error out"=w1515:errorcluster, "pHandle"=w1514:u32, "path out"=w1516:path)  [unwired: 2 in]
            n740 = call "SL2_AD_DLL_Phoibos_ListDeviceModes.vi"("dll path in"=w1516, "dev_type"=w1513, "pHandle"=w1514, "error in"=w1515) -> ("dll path out"=w1510:path, "error out"=w1509:errorcluster)  [unwired: 1 in, 2 out]
          }
          frame #2 {
            n741 = local write "phoib_con?"(TRUE ("phoib_con?")) -> ()
          }
        }
      }
    }
    "phoib_error" <- w1332
  }
  n742 = while {
    tunnel: w2 -> [w1539]
    shift-right: [w1530] -> _
    shift-left: _ -> [w1532]
    shift-right: [w1534] -> _
    shift-left: _ -> [w1533]
    shift-right: [w1527] -> _
    shift-left: -1 ("t") -> [w1531]
    tunnel: w1 -> [w1523]
    stop <- w1535 stop-if-true
    # "watt pilot"
    n743 = Preview Queue Element(queue=w1539, timeout in ms (-1)=w1531) -> (queue out=w1536:refnum<queue>, element=w1541:string)  [unwired: 1 in, 2 out]
    n744 = Match Pattern(string=w1541, regular expression=":") -> (before substring=w1538:string, after substring=w1537:string)  [unwired: 1 in, 2 out]
    n745 = case shown="\"abs\"" w1538 {
      tunnel: w1537 -> [_ _ _ _ w1576 w1607]
      tunnel: w1536 -> [w1546 w1547 w1552 _ w1568 w1613]
      tunnel: [TRUE _ _ _ _ _] -> w1535
      tunnel: [w1543 refnum<visa-resource-name> refnum ("VISA resource name out") w1557 w1565 w1582 w1609] -> w1534
      tunnel: [w1542 w1550 w1556 w1564 w1569 w1608] -> w1530
      tunnel: w1533 -> [w1543 w1551 _ w1567 w1587 w1611]
      tunnel: w1532 -> [w1542 _ w1554 w1566 w1586 w1610]
      tunnel: [0 -1 0 100 0 0] -> w1529
      tunnel: "WP_angle.min" -> [_ _ _ _ w1580 _]
      tunnel: "WP_power.min" -> [_ _ _ _ w1579 _]
      tunnel: "WP_power.max" -> [_ _ _ _ w1578 _]
      tunnel: w1523 -> [_ _ _ _ w1571 _]
      frame "close" {
        n746 = Release Queue(queue=w1546) -> ()  [unwired: 2 in, 3 out]
      }
      frame "release" {
        n747 = Dequeue Element(queue=w1547) -> ()  [unwired: 2 in, 4 out]
        n748 = VISA Close(VISA resource name=w1551) -> (error out=w1550:errorcluster)  [unwired: 1 in]
      }
      frame "init" {
        n749 = Dequeue Element(queue=w1552) -> ()  [unwired: 2 in, 4 out]
        n750 = call <vilib>:"Clear Errors.vi"("error in (no error)"=w1554) -> ("error out"=w1553:errorcluster)  [unwired: 5 in, 1 out]
        n751 = call-poly "VISA Configure Serial Port"("VISA resource name"="WP_VISA", "termination char\n(0xA = '\\n' = LF)"=u8 13 ("termination char\n(0xA = '\\n' = LF)"), "baud rate (9600)"="WP_baud", "error in (no error)"=w1553) -> ("VISA resource name out"=w1557:refnum<visa-resource-name>, "error out"=w1556:errorcluster)  [unwired: 10 in]
      }
      frame "idle", Default {
        n752 = call "read_position.vi"("VISA Refnum in"=w1567, "error in (no error)"=w1566) -> ("VISA Refnum out"=w1565:refnum<visa-resource-name>, "Position"=→"WP_pos.steps":i32, "Moving"=→"Moving":bool, "error out"=w1564:errorcluster)  [unwired: 10 in]
      }
      frame "abs" {
        n753 = Dequeue Element(queue=w1568) -> ()  [unwired: 2 in, 4 out]
        n754 = Match Pattern(string=w1576, regular expression=":") -> (before substring=w1573:string, after substring=w1575:string)  [unwired: 1 in, 2 out]
        n755 = Equal?(x=w1575, y="confirm") -> (x = y?=w1572:bool)
        n756 = Decimal String To Number(string=w1573) -> (number=w1585:i32)  [unwired: 2 in, 1 out]
        n757 = call "move_abosute.vi"("VISA Refnum in"=w1587, "Position"=w1585, "error in (no error)"=w1586) -> ("VISA Refnum out"=w1584:refnum<visa-resource-name>, "error out"=w1583:errorcluster)  [unwired: 11 in]
        n758 = while {
          shift-right: [w1600] -> w1582
          shift-left: w1584 -> [w1605]
          shift-right: [w1601] -> w1570
          shift-left: w1583 -> [w1604]
          tunnel: w1580 -> [w1595]
          tunnel: w1579 -> [w1594]
          tunnel: w1578 -> [w1593]
          stop <- w1602 stop-if-true
          n759 = call "read_position.vi"("VISA Refnum in"=w1605, "error in (no error)"=w1604) -> ("VISA Refnum out"=w1600:refnum<visa-resource-name>, "Position"=w1598:i32, "Moving"=w1599:bool, "error out"=w1601:errorcluster)  [unwired: 10 in]
          n760 = Not(x=w1599) -> (.not. x?=w1603:bool)
          n761 = call "Steps2deg_power.vi"("Max_power"=w1593, "Min_power"=w1594, "Min_angle"=w1595, "Steps"=w1598) -> ("Power"=w1596:dbl, "Deg"=w1597:dbl)  [unwired: 6 in]
          n762 = local write "WP_pos.steps"(w1598) -> ()
          n763 = local write "Moving"(w1599) -> ()
          n764 = Or(x=w1603, y=w1601) -> (x .or. y?=w1602:bool)
          n765 = local write "WP_power"(w1596) -> ()
          n766 = local write "WP_deg"(w1597) -> ()
        }
        n767 = case shown="True" w1572 {
          tunnel: w1571 -> [_ w1591]
          tunnel: w1570 -> [w1588 w1590]
          tunnel: [w1588 w1589] -> w1569
          frame False {
          }
          frame True {
            n768 = Send Notification(notification=TRUE, notifier=w1591, error in (no error)=w1590) -> (error out=w1589:errorcluster)  [unwired: 1 out]
          }
        }
      }
      frame "rel" {
        n769 = Dequeue Element(queue=w1613) -> ()  [unwired: 2 in, 4 out]
        n770 = Decimal String To Number(string=w1607) -> (number=w1606:i32)  [unwired: 2 in, 1 out]
        n771 = call "move_relative.vi"("VISA Refnum in"=w1611, "Position"=w1606, "error in (no error)"=w1610) -> ("VISA Refnum out"=w1609:refnum<visa-resource-name>, "error out"=w1608:errorcluster)  [unwired: 11 in]
      }
    }
    "WP_error" <- w1530
    n772 = Select(t=-1, s=w1530, f=w1529) -> (s? t:f=w1527:i32)
  }
